vi "Interfaz grafica - corriente.vi"() -> ()   [LabVIEW 2024]
uses:
  160620 Optotune Lens Driver 4 Labview package/Hello Optotune Lens (30.06.2015)/Calibration.ctl
  <vilib>/DAQmx/read.llb/DAQmx Read (Analog 1D Wfm NChan NSamp).vi
  <vilib>/Analysis/2dsp.llb/Decimate (single shot, DBL).vi
  <vilib>/Utility/file.llb/Read Delimited Spreadsheet (string).vi
  <vilib>/Instr/_visa.llb/VISA Configure Serial Port (Instr).vi
  <vilib>/DAQmx/create/channels.llb/DAQmx Create Channel (AI-Voltage-Basic).vi
  <vilib>/DAQmx/configure/timing.llb/DAQmx Timing (Sample Clock).vi
  <vilib>/DAQmx/miscellaneous.llb/DAQmx Fill In Error Info.vi
  <vilib>/Waveform/WDTOps.llb/WDT Index Channel DBL.vi
  <vilib>/Analysis/2dsp.llb/Decimate (continuous, DBL).vi
  <vilib>/Utility/file.llb/Write Delimited Spreadsheet (string).vi
  <vilib>/Waveform/WDTOps.llb/WDT Get Waveform Time Array DBL.vi
  <vilib>/Analysis/NI_AALPro.lvlib
panel:
  out "Array 4":string[](array[string])
  out "Array 3":string[](array[string])
  out "Array 2":string[](array[string])
  out "Array":string[](array[string])
  out "Nombre 2":string
  in  "Restablecer Iniciales":bool
  in  "Incremento":dbl=0.1 format="%#_13g"
  out "Potencia derecho":dbl
  out "error out 4":errorcluster
  out "error out 3":errorcluster
  out "error out 2":errorcluster
  in  "Tab Control 3":enum32{"WL", "Video"}(tab)
  out "Waveform length":dbl[][](graph)
  in  "Minimo escala Y":dbl format="%#_13g"
  in  "Maximo escala Y":dbl format="%#_13g"
  in  "Escala autom. Y":u8=1
  in  "Escala autom. X":u8=1
  in  "Maximo escala X":dbl
  in  "Minimo escala X":dbl
  out "VISA resource name out":string
  in  "Tab Control 2":T1(tab)
  in  "DAQmx Physical Channel":tag
  in  "Frecuencia muestreo":i32=20000
  in  "tamaño buffer":i32=1000
  in  "factor decimacion":i32=20
  in  "Ganancia":u16(ring) items=["0.2"=51455, "1"=33023, "10"=49407, "20"=41215, "30"=57599, "40"=37119, "60"=53503, "80"=45311, "120"=61695, "157"=35071, ""=0]
  in  "Potencia inicial lente derecho":dbl(slide) scale=-3.0..3.0
  in  "Potencia inicial lente izquierdo":dbl(slide) scale=-3.0..3.0
  in  "VISA resource name":string="COM11"
  in  "VISA resource name 2":string="COM10"
  out "DPT INICIALES D":dbl
  out "DPT INICIALES I":dbl
  out "Potencia izquierdo":dbl
  in  "error in (no error) 5":errorcluster
  in  "error in (no error) 4":errorcluster
  in  "error in (no error) 3":errorcluster
  in  "error in (no error) 2":errorcluster
  in  "Calibration 4":T2={"Max Current A"=293.0, "Max Current B"=293.0, "UCL A"=300.0, "UCL B"=300.0, "LCL A"=0.0, "LCL B"=0.0} {"Max Current A" format="%#_g mA"; "Max Current B" format="%#_g mA"; "UCL A" format="%#_g mA"; "LCL A" format="%#_g mA"; "UCL B" format="%#_g mA"; "LCL B" format="%#_g mA"}
  out "ID 2":u16
  out "VISA resource name out 2":string
  out "Calibration 3":T2 {"Max Current A" format="%#_g mA"; "Max Current B" format="%#_g mA"; "UCL A" format="%#_g mA"; "LCL A" format="%#_g mA"; "UCL B" format="%#_g mA"; "LCL B" format="%#_g mA"}
  out "OK 2":bool
  out "Data 2":string
  out "Command to Port 2":string
  in  "Cola tipo 2":dbl[](array[numeric])
  in  "Tamaño ventana WL":i32=60
  in  "Limite inferior WL":dbl=25.0 format="%#_13g"
  in  "Limite superior WL":dbl=50.0
  out "number":u32
  in  "Calibration":T2={"Max Current A"=293.0, "Max Current B"=293.0, "UCL A"=300.0, "UCL B"=300.0, "LCL A"=0.0, "LCL B"=0.0} {"Max Current A" format="%#_g mA"; "Max Current B" format="%#_g mA"; "UCL A" format="%#_g mA"; "LCL A" format="%#_g mA"; "UCL B" format="%#_g mA"; "LCL B" format="%#_g mA"}
  out "ID":u16
  out "Calibration 2":T2 {"Max Current A" format="%#_g mA"; "Max Current B" format="%#_g mA"; "UCL A" format="%#_g mA"; "LCL A" format="%#_g mA"; "UCL B" format="%#_g mA"; "LCL B" format="%#_g mA"}
  out "OK":bool
  out "Data":string
  out "Command to Port":string
  in  "DPT dif.":dbl
  out "error out":errorcluster
  in  "error in (no error)":errorcluster
  in  "WL":dbl
  in  "Cola tipo":dbl[](array[numeric])
  out "T button?":bool
  in  "Elegir menu Exp":bool
  in  "Elegir menu":bool
  out "path":path
  in  "Iniciar experimento":bool
  in  "Parar adquisicion":bool
  out "Enfermedad visual":string
  out "Edad":string
  out "Nombre":string
  out "Cedula":string
  in  "Carpeta":path=path "C:/Users/TGM1603/Documents/LabVIEW Data/Experimentos electrodos"
  in  "?":bool
  in  "Menu Principal":u16(ring) items=["Visualizacion general ", "Llevar a cabo un experimento", "Ajustar potencia inicial lentes"]
  in  "Menu experimentos":u16(ring) items=["Experimento 1", "Experimento 2", "Experimento 3", "Experimento 4"]
  in  "Tab Control":enum32{"Señal EMG", "Potencia "}(tab)
  out "Senal EMG":waveform(dbl)[](graph)
  in  "Escala automatica Y":u8
  in  "Escala automatica X":u8=1
  in  "X Scale.Range:Increment":dbl
  in  "X Scale.Range:Minimum":dbl
  in  "X Scale.Range:Maximum":dbl
  in  "Y Scale.Range:Minimum":dbl=-5.0
  in  "Y Scale.Range:Maximum":dbl=5.0
  in  "Escala Y min":dbl
  in  "Escala Y max":dbl
  in  "Auto scale Y":u8=1
  in  "Escala X max":dbl
  in  "Escala X min":dbl
  out "Potencia Optica":dbl[](graph)
  in  "Auto scale X":u8=1
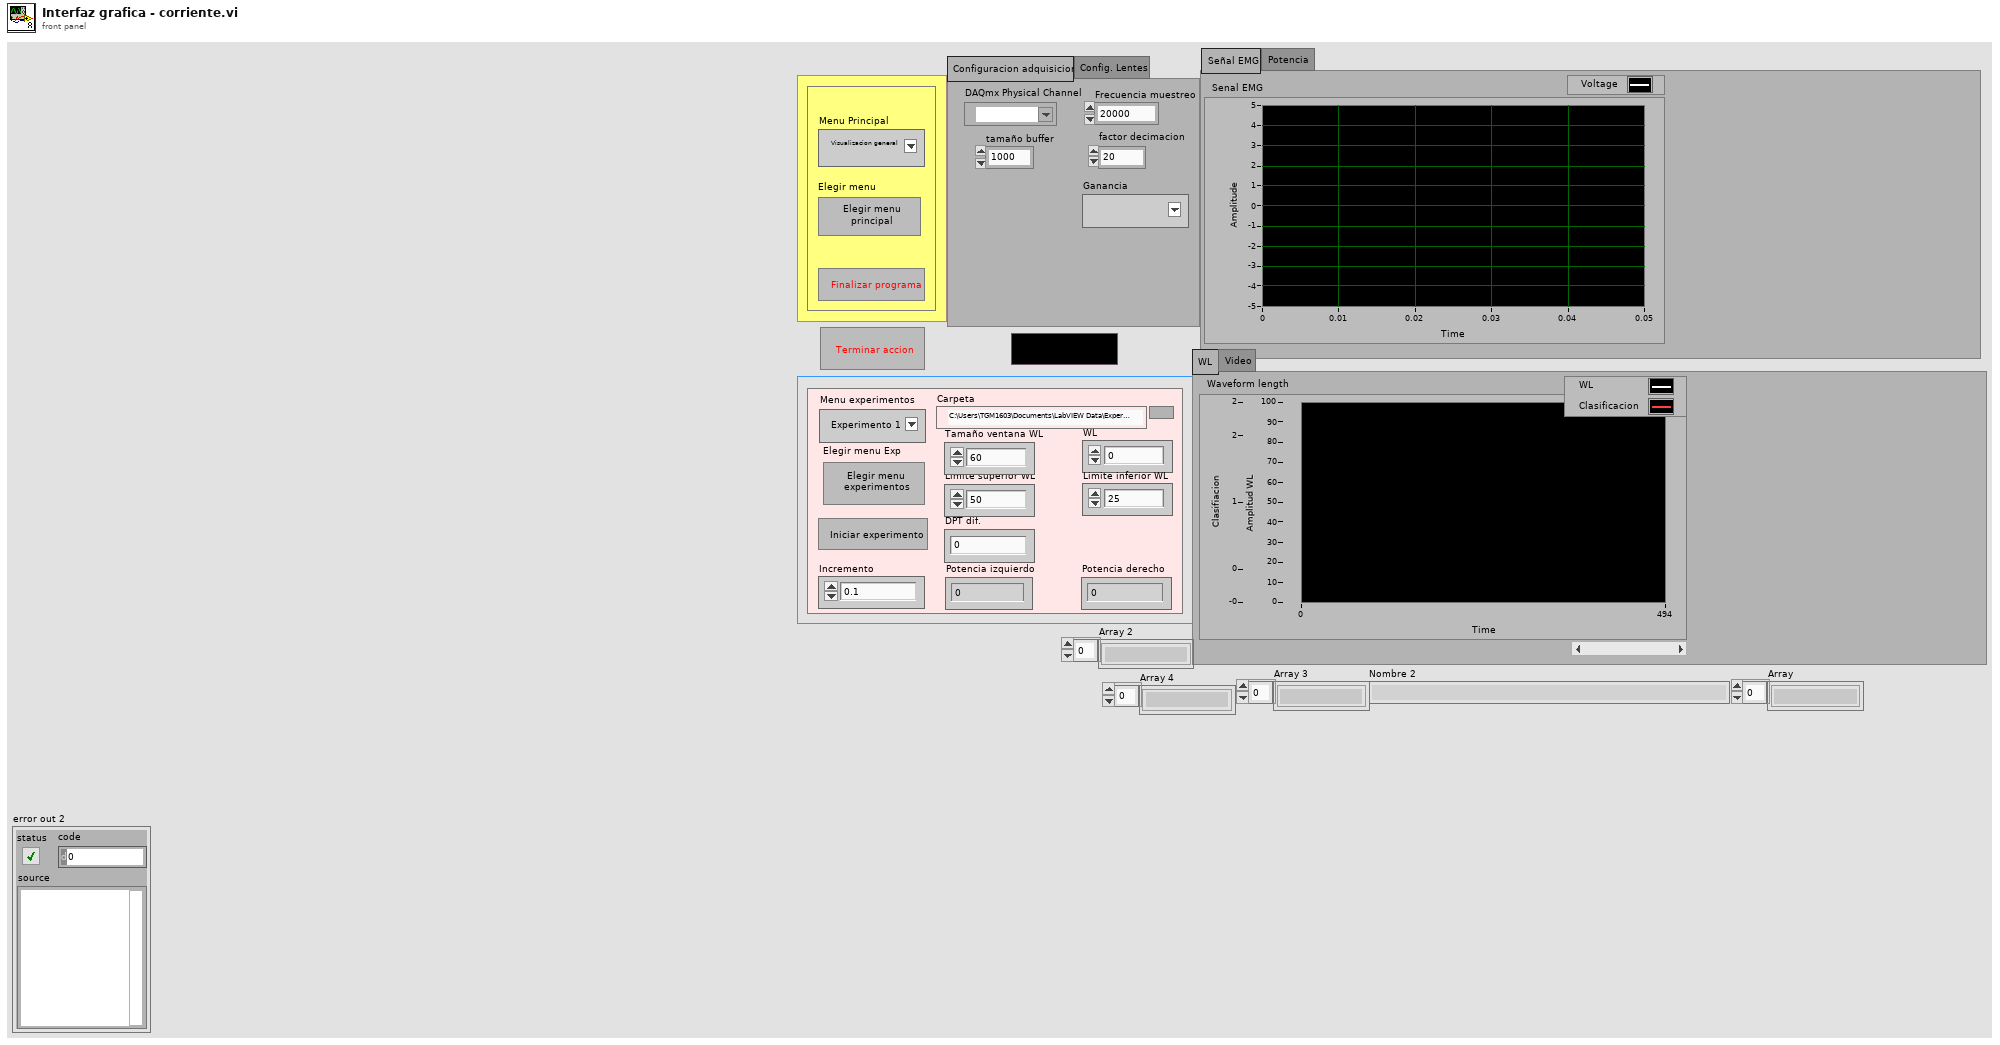
[diagram p1: front panel]
types:
  T1 = enum32{"Configuracion adquisicion", "Config. Lentes"}
  T2 = typedef "Calibration.ctl" = cluster{"Max Current A":dbl, "Max Current B":dbl, "UCL A":dbl, "UCL B":dbl, "LCL A":dbl, "LCL B":dbl}
  T3 = enum16{"Left Button", "Center Button", "Right Button", "Window Close"}
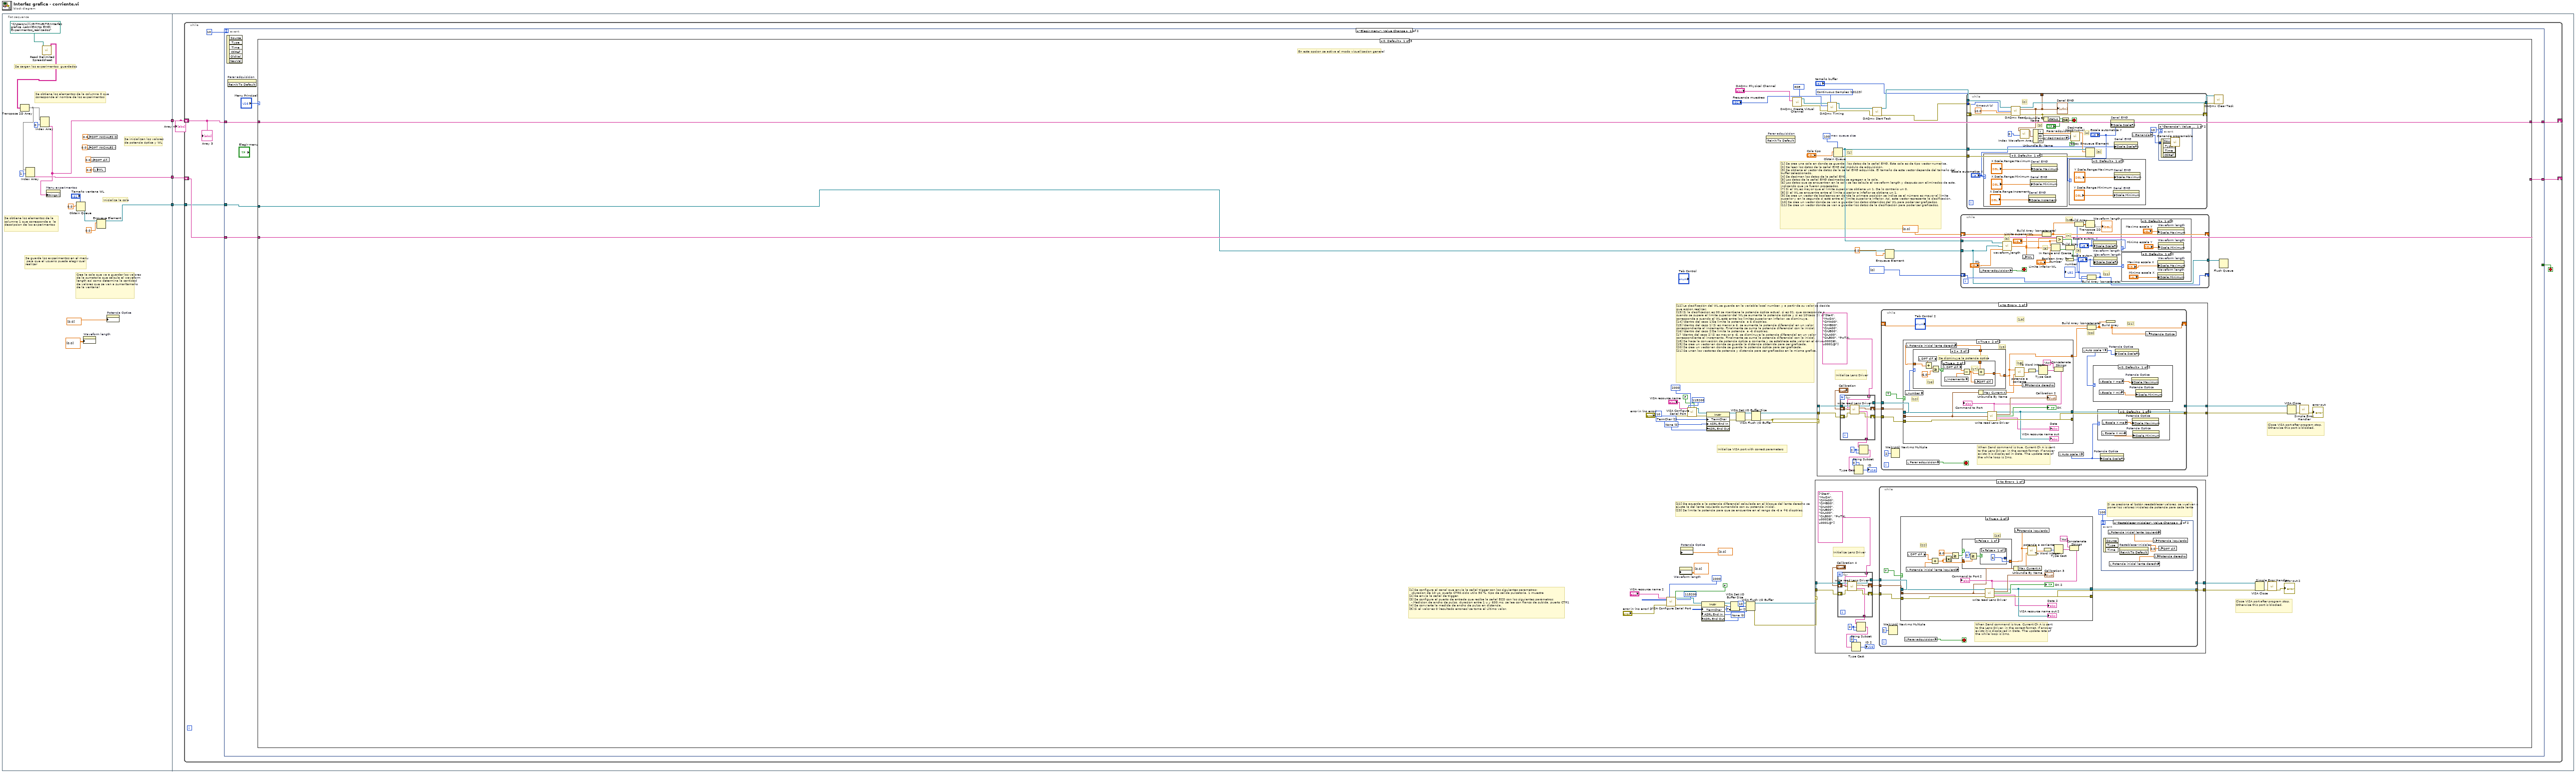
[diagram p0: block diagram]
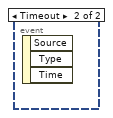
[diagram p2: hidden frame]
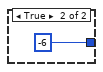
[diagram p4: hidden frame]
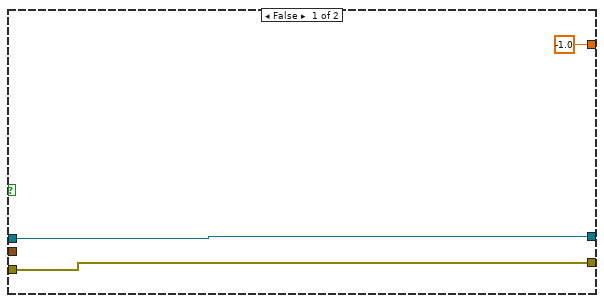
[diagram p9: hidden frame]
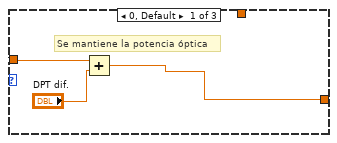
[diagram p10: hidden frame]
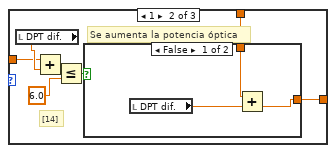
[diagram p11: hidden frame]
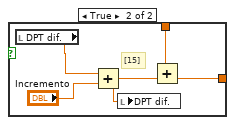
[diagram p12: hidden frame]
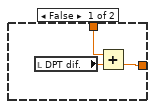
[diagram p13: hidden frame]
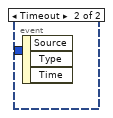
[diagram p17: hidden frame]
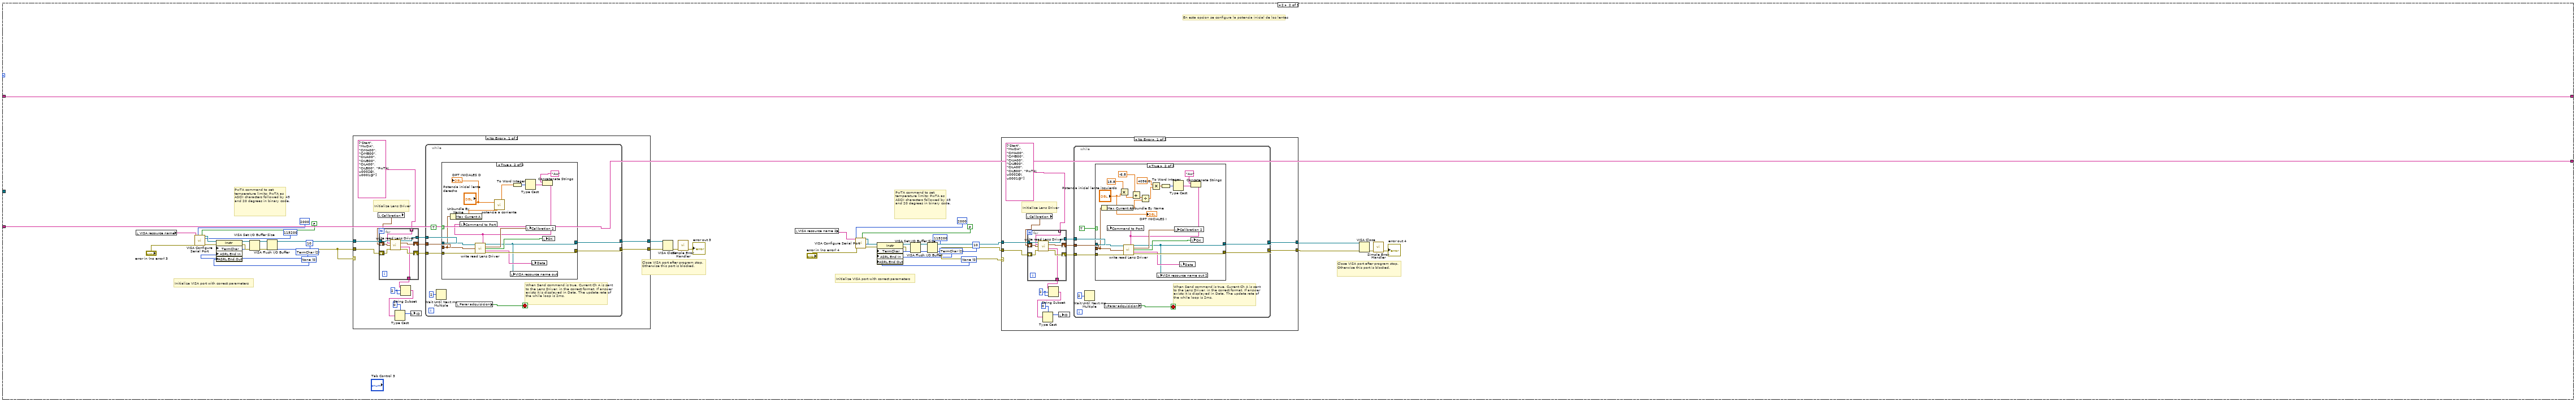
[diagram p20: hidden frame]
diagram:
  n1 = flat-sequence {
    tunnel: [w18] -> w3
    tunnel: [w15] -> w2
    tunnel: [w10] -> w1
    tunnel: w3 -> [w22]
    tunnel: w2 -> [w24]
    tunnel: w1 -> [w23]
    frame #0 {
      # "Se inicializan los valores\nde potencia óptica y WL"
      # "Inicializa la cola"
      # "Crea la cola que va a guardar los valores de la sumatoria que calcula el waveform length así como determina la cantidad de valores que se van a sumar(tamaño de la ventana)"
      # "Se obtiene los elementos de la columna 1 que corresponde a  la descripcion de los experimentos"
      # "Se obtiene los elementos de la columna 0 que corresponde al nombre de los experimentos"
      # "Se guarda los experimentos en el menu\n para que el usuario pueda elegir cual \nrealizar"
      # "Se cargan los experimentos  guardados"
      n2 = call-poly <vilib>:"Read Delimited Spreadsheet.vi"("file path (dialog if empty)"=path "C:/Users/willi/GITHUB/TG/Interfaz grafica -LabVIEW/No EMG/Experimentos_realizados") -> ("all rows"=w19:string[][])  [unwired: 9 in, 5 out]
      n3 = Transpose 2D Array(2D array=w19) -> (transposed array=w16:string[][])
      n4 = Index Array(array=w16, index (row)=1) -> (element=w15:string[])  [unwired: 1 in]
      n5 = Index Array(array=w16, index (row)=0) -> (element=w18:string[])  [unwired: 1 in]
      n6 = property on="Menu experimentos" class="Ring (strict)"("Strings []"=w18) -> ()  [unwired: 2 in, 2 out]
      n7 = Obtain Queue(max queue size (-1, unlimited)="Tamaño ventana WL", element data type=0.0) -> (queue out=w13:refnum<queue>)  [unwired: 3 in, 2 out]
      n8 = property on="Waveform length" class="WFChart (strict)"("History Data"=dbl[][] [[0.0]]) -> ()  [unwired: 2 in, 2 out]
      n9 = local write "DPT INICIALES D"(0.0 ("DPT INIT.1")) -> ()
      n10 = local write "DPT INICIALES I"(0.0 ("DPT INIT.2")) -> ()
      n11 = local write "DPT dif."(0.0 ("WL")) -> ()
      n12 = local write "WL"(0.0 ("WL")) -> ()
      n13 = Enqueue Element(queue=w13, element=0.0) -> (queue out=w10:refnum<queue>)  [unwired: 2 in, 2 out]
      n14 = property on="Potencia Optica" class="WFChart (strict)"("History Data"=dbl[] [0.0]) -> ()  [unwired: 2 in, 2 out]
    }
    frame #1 {
      n15 = while {
        shift-right: [w30] -> _
        shift-left: w22 -> [w31]
        shift-right: [w28] -> _
        shift-left: w24 -> [w29]
        tunnel: w23 -> [w27]
        stop <- w26 stop-if-true
        n16 = event shown="[0] \"Elegir menu\": Value Change" {
          selector: _ -> [_ _]
          dyn-events: _ -> [_ _]
          timeout: 10 -> [_ _]
          tunnel: w31 -> [w37 w978]
          tunnel: [w36 w978] -> w30
          tunnel: w29 -> [w35 w977]
          tunnel: [w34 w977] -> w28
          tunnel: w27 -> [w32 _]
          tunnel: [_ "?"] -> w26
          event "Elegir menu": Value Change {
            n17 = event-data() -> ()  [unwired: 1 in, 6 out]
            n18 = invoke on="Parar adquisicion" class="Bool (strict)" method="Reinit To Default"() -> ()  [unwired: 3 in, 3 out]
            n19 = case shown="0, Default" "Menu Principal" {
              tunnel: w37 -> [w104 w357 w477]
              tunnel: [w104 w357 w476] -> w36
              tunnel: w35 -> [w103 w356 w474]
              tunnel: [w103 w356 w473] -> w34
              tunnel: w32 -> [w93 _ w464]
              frame 0, Default {
                w38 = 10123 items=["Finite Samples"=10178, "Continuous Samples"=10123, "Hardware Timed Single Point"=12522] ("sample mode")
                w39 = 10083 items=["Default"=-1, "RSE"=10083, "NRSE"=10078, "Differential"=10106, "Pseudodifferential"=12529] ("input terminal configuration")
                w61 = u16 0 items=["None", "Last Bit", "TermChar", "Break"] ("Serial Settings:End Mode for Writes")
                w60 = u16 2 items=["None", "Last Bit", "TermChar"] ("Serial Settings:End Mode for Reads")
                w83 = u16 0 items=["None", "Last Bit", "TermChar", "Break"] ("Serial Settings:End Mode for Writes")
                w84 = u16 2 items=["None", "Last Bit", "TermChar"] ("Serial Settings:End Mode for Reads")
                w97 = 100  # max queue size
                # "[22] De acuerda a la potencia diferencial calculada en el bloque del lente derecho se ajusta la del lente izquierdo sumandola con su potencia inicial.\n[23] Se limita la potencia para que se encuentre en el rango de -6 a +6 dioptrías."
                # "[12] La clasificación del WL se guarda en la variable local number, y a partir de su valor se decide que accion realizar.\n[13] Si la clasificacion es 00 se mantiene la potencia óptica actual, si es 01, que corresponde a cuando se supera el limite superior del WL,se aumenta la potencia óptica y si es 10(caso 2), que corresponde a cuando el WL está entre los limites superior en inferior, se disminuye. \n[14] (dentro del caso 1)Se limita la potencia  a 6 dioptrías. \n[15] (dentro del caso 1) Si es menor a 6, se aumenta la potencia diferencial en un valor correspondiente al incremento. Finalmente se suma la potencia diferencial con la inicial.\n[16] (dentro del caso 2)Se limita la potencia  a -6 dioptrías.\n[17 (dentro del caso 2) Si es mayor a -6, se disminuye la potencia diferencial en un valor correspondiente al incremento. Finalmente se suma la potencia diferencial con la inicial.\n[18] Se hace la conversión de potencia óptica a corriente y se establece este valor en el driver.\n[19] Se crea un vector en donde se guarda la distancia obtenida para ser graficada.\n[20] Se crea un vector en donde se guarda la potencia óptica para ser graficada.\n[21] Se unen los vectores de potencia y distancia para ser graficados en la misma grafica."
                # "[1] Se crea una cola en donde se guardan los datos de la señal EMG. Esta cola es de tipo vector numerica.\n[2] Se leen los datos de la señal EMG del módulo de adquisición. \n[3] Se obtiene el vector de datos de la señal EMG adquirida. El tamaño de este vector depende del tamaño del buffer seleccionado.\n[4] Se deciman los datos de la señal EMG.\n[5] Los datos de la señal EMG decimados se agregan a la cola.\n[6] Los datos que se encuentran en la cola se les calcula el waveform length y después son eliminados de esta, indicando que ya fueron procesados. \n[7] Si el WL es mayor que el limite superior se obtiene un 1. De lo contrario un 0.\n[8] Si el WL se encuentra entre el límite superior e infefior se obtiene un 1.\n[9] Se crea un vector de booleanos en donde la primera posición se indica se el número es mayor al límite superior y en la segunda si está entre el  limite superior e inferior. Así, este vector representa la clasificación.\n[10] Se crea un vector donde se van a guardar los datos obtenidos del WL para poder ser graficados.\n[11] Se crea un vector donde se van a guardar los datos de la clasificación para poder ser graficados."
                # "[1]"
                # "En esta opcion se activa el modo visualizacion general"
                # "Close VISA port after program stop. Otherwise this port is blocked."
                # "[1] Se configura el canal que envía la señal trigger con los siguientes parametros:\n  -duracion de 10 us, puerto CTR0,ciclo utilo 50 %, tipo de salida pulsatoria, 1 muestra \n[2] Se envía la señal de trigger.\n[3] Se configura el puerto de entrada que recibe la señal ECO con los siguientes parámetros:\n  - Medicion de ancho de pulso, duracion entre 1 u y 600 ms, se lee con flanco de subida, puerto CTR1\n[4] Se convierte la medida de ancho de pulso en distancia.\n[5] Si el valor es 0 (resultado erroneo) se toma el último valor."
                # "Close VISA port after program stop. Otherwise this port is blocked."
                # "Initialize VISA port with correct parameters"
                n20 = call-poly "VISA Configure Serial Port"("VISA resource name"="VISA resource name 2", "timeout (10sec)"=u32 2000, "Enable Termination\nChar (T)"=FALSE ("Enable Termination\nChar (T)"), "baud rate (9600)"=u32 115200, "error in (no error)"="error in (no error) 2") -> ("VISA resource name out"=w56:refnum<visa-resource-name>, "error out"=w58:errorcluster)  [unwired: 9 in]
                n21 = property on="Waveform length" class="WFChart (strict)"("History Data"=dbl[][] [[0.0]]) -> ()  [unwired: 2 in, 2 out]
                n22 = property on="Potencia Optica" class="WFChart (strict)"("History Data"=dbl[] [0.0]) -> ()  [unwired: 2 in, 2 out]
                n23 = call-poly "VISA Configure Serial Port"("VISA resource name"="VISA resource name", "timeout (10sec)"=u32 2000, "Enable Termination\nChar (T)"=FALSE ("Enable Termination\nChar (T)"), "baud rate (9600)"=u32 115200, "error in (no error)"="error in (no error)") -> ("VISA resource name out"=w88:refnum<visa-resource-name>, "error out"=w86:errorcluster)  [unwired: 9 in]
                n24 = property class="Instr"(reference=w56, error in=w58, "TermChar"=u8 10 ("Message Based Settings:Termination Character"), "ASRL End In"=w60, "ASRL End Out"=w61) -> (reference out=w57:refnum<visa-resource-name>, error out=w59:errorcluster)
                n25 = property class="Instr"(reference=w88, error in=w86, "TermChar"=u8 10 ("Message Based Settings:Termination Character"), "ASRL End In"=w84, "ASRL End Out"=w83) -> (reference out=w87:refnum<visa-resource-name>, error out=w85:errorcluster)
                n26 = VISA Set I/O Buffer Size(VISA resource name=w57, error in (no error)=w59) -> (VISA resource name out=w64:refnum<visa-resource-name>, error out=w65:errorcluster)  [unwired: 2 in]
                n27 = VISA Set I/O Buffer Size(VISA resource name=w87, error in (no error)=w85) -> (VISA resource name out=w80:refnum<visa-resource-name>, error out=w79:errorcluster)  [unwired: 2 in]
                n28 = VISA Flush I/O Buffer(VISA resource name=w64, error in (no error)=w65) -> (VISA resource name out=w50:refnum<visa-resource-name>, error out=w51:errorcluster)  [unwired: 1 in]
                n29 = VISA Flush I/O Buffer(VISA resource name=w80, error in (no error)=w79) -> (VISA resource name out=w78:refnum<visa-resource-name>, error out=w73:errorcluster)  [unwired: 1 in]
                n30 = invoke on="Parar adquisicion" class="Bool (strict)" method="Reinit To Default"() -> ()  [unwired: 3 in, 3 out]
                n31 = call-poly <vilib>:"DAQmx Create Virtual Channel.vi"("input terminal configuration"=w39, "physical channels"="DAQmx Physical Channel") -> ("task out"=w45:refnum<k21>, "error out"=w44:errorcluster)  [unwired: 12 in]
                n32 = case shown="No Error" w51 {
                  tunnel: w51 -> [w118 w169]
                  tunnel: w50 -> [w117 w170]
                  tunnel: [w116 w169] -> w46
                  tunnel: [w115 w170] -> w47
                  frame No Error {
                    w113 = 2 ("length (rest)")
                    # "Initialize Lens Driver"
                    n33 = for {
                      tunnel: w117 -> [w167]
                      tunnel: [w164] -> w107
                      tunnel: string[] ["Start", "MwDA", "CrMA00", "CrMB00", "CrUA00", "CrUB00", "CrLA00", "CrLB00", "PwTA\u0002Ð\u0001@"] -> [w162] mode=indexing
                      tunnel: [w161] -> w106
                      shift-right: [w165] -> w108
                      shift-left: "Calibration 4" -> [w166]
                      shift-right: [w163] -> w109
                      shift-left: w118 -> [w168]
                      n34 = call "write read Lens Driver.vi"("VISA resource name"=w167, "command"=w162, "Calibration"=w166, "error in (no error)"=w168) -> ("VISA resource name out"=w164:refnum<visa-resource-name>, "Calibration 2"=w165:T2, "Data"=w161:string, "error out"=w163:errorcluster)  [unwired: 4 in, 4 out]
                    }
                    n35 = String Subset(string=w106, offset (0)=w113, length (rest)=w113) -> (substring=w111:string)
                    n36 = Type Cast(type=u16 0 ("length (rest)"), x=w111) -> (*(type *) &x=→"ID 2":u16)
                    n37 = while {
                      tunnel: [w121] -> w116
                      tunnel: [w122] -> w115
                      tunnel: w109 -> [w127]
                      tunnel: w108 -> [w126]
                      tunnel: w107 -> [w125]
                      stop <- w120 stop-if-true
                      # "Si se presiona el botón reestablecer valores, se vuelven a poner los valores iniciales de potencia para cada lente"
                      # "When Send command is true, Current Ch A is sent to the Lens Driver, in the correct format. If answer exists it is displayed in Data. The update rate of the while loop is 2ms."
                      n38 = Wait Until Next ms Multiple(millisecond multiple=u32 2) -> ()  [unwired: 1 out]
                      n39 = case shown="True" TRUE ("Send command") {
                        tunnel: [w132 w153] -> w121
                        tunnel: w127 -> [w132 w152]
                        tunnel: w126 -> [_ w134]
                        tunnel: w125 -> [w131 w151]
                        tunnel: [w131 w148] -> w122
                        frame False {
                        }
                        frame True {
                          # "[23]"
                          # "[22]"
                          n40 = local read "Potencia inicial lente izquierdo"() -> (w142:dbl)
                          n41 = local read "DPT dif."() -> (w143:dbl)
                          n42 = Add(x=w143, y=w142) -> (x+y=w138:dbl)
                          n43 = Absolute Value(x=w138) -> (abs(x)=w140:dbl)
                          n44 = Greater Or Equal?(x=6.0, y=w140) -> (x >= y?=w141:bool)
                          n45 = case shown="False" w141 {
                            tunnel: w138 -> [w156 w160]
                            tunnel: [w154 w160] -> w136
                            frame False {
                              n46 = Greater Or Equal?(x=u16 0, y=w156) -> (x >= y?=w157:bool)
                              n47 = case shown="False" w157 {
                                tunnel: [i16 6 ("x") i16 -6 ("x")] -> w154
                                frame False {
                                }
                                frame True {
                                }
                              }
                            }
                            frame True {
                            }
                          }
                          n48 = Unbundle By Name(w134) -> ("Max Current A"=w135:dbl)
                          n49 = local write "Potencia izquierdo"(w136) -> ()
                          n50 = call "potencia a corriente.vi"("Max current A"=w135, "Potencia"=w136) -> ("Corriente"=w137:dbl)
                          n51 = To Word Integer(number=w137) -> (16bit integer=w146:i16)
                          n52 = Type Cast(x=w146) -> (*(type *) &x=w145:string)  [unwired: 1 in]
                          n53 = Concatenate Strings("Aw", w145) -> (w144:string)
                          "Command to Port 2" <- w144
                          n54 = call "write read Lens Driver.vi"("VISA resource name"=w151, "command"=w144, "Calibration"=w134, "error in (no error)"=w152) -> ("VISA resource name out"=w148:refnum<visa-resource-name>, "Calibration 2"=→"Calibration 3":T2, "OK"=→"OK 2":bool, "Data"=→"Data 2":string, "error out"=w153:errorcluster)  [unwired: 4 in, 3 out]
                          "VISA resource name out 2" <- w148
                        }
                      }
                      n55 = local read "Parar adquisicion"() -> (w120:bool)
                      n56 = event shown="[0] \"Restablecer Iniciales\": Value Change" {
                        selector: _ -> [_ _]
                        dyn-events: _ -> [_ _]
                        timeout: 100 -> [_ _]
                        event "Restablecer Iniciales": Value Change {
                          n57 = event-data() -> ()  [unwired: 1 in, 3 out]
                          n58 = local read "Potencia inicial lente izquierdo"() -> (w128:dbl)
                          n59 = local read "Potencia inicial lente derecho"() -> (w129:dbl)
                          n60 = invoke on="Restablecer Iniciales" class="Bool" method="Reinit To Default"() -> ()  [unwired: 3 in, 3 out]
                          n61 = local write "Potencia izquierdo"(w128) -> ()
                          n62 = local write "Potencia derecho"(w129) -> ()
                          n63 = local write "DPT dif."(0.0 ("DPT dif.")) -> ()
                        }
                        event Timeout {
                          n64 = event-data() -> ()  [unwired: 1 in, 3 out]
                        }
                      }
                    }
                  }
                  frame Error {
                  }
                }
                n65 = case shown="No Error" w73 {
                  tunnel: w73 -> [w184 w263]
                  tunnel: w78 -> [w183 w264]
                  tunnel: [w182 w263] -> w76
                  tunnel: [w181 w264] -> w74
                  frame No Error {
                    w179 = 2 ("length (rest)")
                    # "Initialize Lens Driver"
                    n66 = for {
                      tunnel: w183 -> [w261]
                      tunnel: [w258] -> w173
                      tunnel: string[] ["Start", "MwDA", "CrMA00", "CrMB00", "CrUA00", "CrUB00", "CrLA00", "CrLB00", "PwTA\u0002Ð\u0001@"] -> [w256] mode=indexing
                      tunnel: [w255] -> w172
                      shift-right: [w259] -> w174
                      shift-left: "Calibration" -> [w260]
                      shift-right: [w257] -> w175
                      shift-left: w184 -> [w262]
                      n67 = call "write read Lens Driver.vi"("VISA resource name"=w261, "command"=w256, "Calibration"=w260, "error in (no error)"=w262) -> ("VISA resource name out"=w258:refnum<visa-resource-name>, "Calibration 2"=w259:T2, "Data"=w255:string, "error out"=w257:errorcluster)  [unwired: 4 in, 4 out]
                    }
                    n68 = String Subset(string=w172, offset (0)=w179, length (rest)=w179) -> (substring=w177:string)
                    n69 = Type Cast(type=u16 0 ("length (rest)"), x=w177) -> (*(type *) &x=→"ID":u16)
                    n70 = while {
                      tunnel: [w191] -> w182
                      tunnel: [w192] -> w181
                      tunnel: w175 -> [w197]
                      tunnel: w174 -> [w196]
                      tunnel: w173 -> [w195]
                      shift-right: [w185] -> _
                      shift-left: _ -> [w187]
                      stop <- w190 stop-if-true
                      # "[21]"
                      # "[20]"
                      # "[19]"
                      # "When Send command is true, Current Ch A is sent to the Lens Driver, in the correct format. If answer exists it is displayed in Data. The update rate of the while loop is 2ms."
                      n71 = Wait Until Next ms Multiple(millisecond multiple=u32 2) -> ()  [unwired: 1 out]
                      n72 = case shown="True" TRUE ("Send command") {
                        tunnel: [w204 w221] -> w191
                        tunnel: w197 -> [w204 w220]
                        tunnel: w196 -> [_ w207]
                        tunnel: w195 -> [w203 w219]
                        tunnel: [w203 w216] -> w192
                        tunnel: [-1.0 ("DPT") w209] -> w186
                        frame False {
                        }
                        frame True {
                          # "[18]"
                          # "[13]"
                          # "[12]"
                          n73 = local read "number"() -> (w211:u32)
                          n74 = local read "Potencia inicial lente derecho"() -> (w210:dbl)
                          n75 = case shown="2" w211 {
                            tunnel: [w223 w231 w246] -> w209
                            tunnel: w210 -> [w224 w226 w241]
                            tunnel: w210 -> [_ w225 w240]
                            frame 0, Default {
                              # "Se mantiene la potencia óptica"
                              n76 = Add(x=w224, y="DPT dif.") -> (x+y=w223:dbl)
                            }
                            frame 1 {
                              # "[14]"
                              # "Se aumenta la potencia óptica"
                              n77 = local read "DPT dif."() -> (w227:dbl)
                              n78 = Add(x=w226, y=w227) -> (x+y=w228:dbl)
                              n79 = Less Or Equal?(x=w228, y=6.0) -> (x <= y?=w230:bool)
                              n80 = case shown="False" w230 {
                                tunnel: [w233 w236] -> w231
                                tunnel: w225 -> [w232 w235]
                                frame False {
                                n81 = local read "DPT dif."() -> (w234:dbl)
                                n82 = Add(x=w232, y=w234) -> (x+y=w233:dbl)
                                }
                                frame True {
                                # "[15]"
                                n83 = local read "DPT dif."() -> (w237:dbl)
                                n84 = Add(x=w237, y="Incremento") -> (x+y=w238:dbl)
                                n85 = local write "DPT dif."(w238) -> ()
                                n86 = Add(x=w235, y=w238) -> (x+y=w236:dbl)
                                }
                              }
                            }
                            frame 2 {
                              # "[16]"
                              # "Se disminuye la potencia óptica"
                              n87 = local read "DPT dif."() -> (w245:dbl)
                              n88 = Add(x=w245, y=w241) -> (x+y=w242:dbl)
                              n89 = Greater Or Equal?(x=w242, y=-6.0) -> (x >= y?=w243:bool)
                              n90 = case shown="True" w243 {
                                tunnel: [w248 w252] -> w246
                                tunnel: w240 -> [w247 w251]
                                frame False {
                                n91 = local read "DPT dif."() -> (w249:dbl)
                                n92 = Add(x=w247, y=w249) -> (x+y=w248:dbl)
                                }
                                frame True {
                                # "[17]"
                                n93 = local read "DPT dif."() -> (w254:dbl)
                                n94 = local read "Incremento"() -> (w250:dbl)
                                n95 = Subtract(x=w254, y=w250) -> (x-y=w253:dbl)
                                n96 = local write "DPT dif."(w253) -> ()
                                n97 = Add(x=w251, y=w253) -> (x+y=w252:dbl)
                                }
                              }
                            }
                          }
                          n98 = Unbundle By Name(w207) -> ("Max Current A"=w206:dbl)
                          n99 = call "potencia a corriente.vi"("Max current A"=w206, "Potencia"=w209) -> ("Corriente"=w208:dbl)
                          n100 = local write "Potencia derecho"(w209) -> ()
                          n101 = To Word Integer(number=w208) -> (16bit integer=w214:i16)
                          n102 = Type Cast(x=w214) -> (*(type *) &x=w213:string)  [unwired: 1 in]
                          n103 = Concatenate Strings("Aw", w213) -> (w212:string)
                          "Command to Port" <- w212
                          n104 = call "write read Lens Driver.vi"("VISA resource name"=w219, "command"=w212, "Calibration"=w207, "error in (no error)"=w220) -> ("VISA resource name out"=w216:refnum<visa-resource-name>, "Calibration 2"=→"Calibration 2":T2, "OK"=→"OK":bool, "Data"=→"Data":string, "error out"=w221:errorcluster)  [unwired: 4 in, 3 out]
                          "VISA resource name out" <- w216
                        }
                      }
                      n105 = local read "Parar adquisicion"() -> (w190:bool)
                      n106 = local read "Auto scale X"() -> (w188:u8)
                      n107 = local read "Auto scale Y"() -> (w189:u8)
                      n108 = Build Array (concatenate)(w187, w186) -> (w185:dbl[])
                      n109 = case shown="0, Default" w189 {
                        frame 0, Default {
                          n110 = local read "Escala Y max"() -> (w201:dbl)
                          n111 = local read "Escala Y min"() -> (w200:dbl)
                          n112 = property on="Potencia Optica" class="WFChart (strict)"("YScale.Maximum"=w201) -> ()  [unwired: 2 in, 2 out]
                          n113 = property on="Potencia Optica" class="WFChart (strict)"("YScale.Minimum"=w200) -> ()  [unwired: 2 in, 2 out]
                        }
                        frame 1 {
                        }
                      }
                      n114 = case shown="0, Default" w188 {
                        frame 0, Default {
                          n115 = local read "Escala X min"() -> (w198:dbl)
                          n116 = local read "Escala X max"() -> (w199:dbl)
                          n117 = property on="Potencia Optica" class="WFChart (strict)"("XScale.Maximum"=w199) -> ()  [unwired: 2 in, 2 out]
                          n118 = property on="Potencia Optica" class="WFChart (strict)"("XScale.Minimum"=w198) -> ()  [unwired: 2 in, 2 out]
                        }
                        frame 1 {
                        }
                      }
                      n119 = property on="Potencia Optica" class="WFChart (strict)"("XScale.ScaleFit"=w188) -> ()  [unwired: 2 in, 2 out]
                      n120 = Build Array(w185) -> ()  [unwired: 1 out]
                      n121 = property on="Potencia Optica" class="WFChart (strict)"("YScale.ScaleFit"=w189) -> ()  [unwired: 2 in, 2 out]
                      n122 = local write "Potencia Optica"(w185) -> ()
                    }
                  }
                  frame Error {
                  }
                }
                n123 = call-poly <vilib>:"DAQmx Timing.vi"("task/channels in"=w45, "sample mode"=w38, "rate"="Frecuencia muestreo", "error in"=w44) -> ("task out"=w43:refnum<k21>, "error out"=w42:errorcluster)  [unwired: 10 in]
                n124 = Obtain Queue(max queue size (-1, unlimited)=w97, element data type="Cola tipo") -> (queue out=w94:refnum<queue>, error out=w95:errorcluster)  [unwired: 3 in, 1 out]
                n125 = call <vilib>:"DAQmx Start Task.vi"("task/channels in"=w43, "error in"=w42) -> ("task out"=w102:refnum<k21>, "error out"=w101:errorcluster)  [unwired: 12 in]
                n126 = Enqueue Element(queue=w93, element=0.0) -> (queue out=w70:refnum<queue>)  [unwired: 2 in, 2 out]
                n127 = while {
                  tunnel: w70 -> [w266]
                  tunnel: w94 -> [w283]
                  shift-right: [w269] -> _
                  shift-left: dbl[] [0.0] -> [w280]
                  shift-right: [w268] -> _
                  shift-left: u32[] [0] -> [w270]
                  tunnel: [w266] -> w68
                  stop <- w281 stop-if-true
                  # "[11]"
                  # "[10]"
                  # "[9]"
                  # "[8]"
                  # "[7]"
                  # "[6]"
                  n128 = local read "Parar adquisicion"() -> (w281:bool)
                  n129 = call "waveform_length.vi"("WL"="WL", "Cola WL"=w266, "Datos entrada"=w283) -> ("WL 2"=w278:dbl)
                  n130 = local write "WL"(w278) -> ()
                  n131 = Build Array (concatenate)(w280, w278) -> (w269:dbl[])
                  n132 = In Range and Coerce(upper limit="Limite superior WL", x=w278, lower limit="Limite inferior WL") -> (In Range?=w276:bool)  [unwired: 1 out]
                  n133 = Greater?(x=w278, y="Limite superior WL") -> (0:w277:bool)
                  n134 = Build Array(w277, w276) -> (w275:bool[])
                  n135 = Boolean Array To Number(Boolean array=w275) -> (number=w271:u32)
                  "number" <- w271
                  n136 = Build Array (concatenate)(w270, w271) -> (w268:u32[])
                  n137 = Build Array(w269, w268) -> (w267:dbl[][])
                  n138 = Transpose 2D Array(2D array=w267) -> (transposed array=→"Waveform length":dbl[][])
                  n139 = property on="Waveform length" class="WFChart (strict)"("YScale.ScaleFit"="Escala autom. Y") -> ()  [unwired: 2 in, 2 out]
                  n140 = property on="Waveform length" class="WFChart (strict)"("XScale.ScaleFit"="Escala autom. X") -> ()  [unwired: 2 in, 2 out]
                  n141 = case shown="0, Default" "Escala autom. Y" {
                    frame 0, Default {
                      n142 = property on="Waveform length" class="WFChart (strict)"("YScale.Maximum"="Maximo escala Y") -> ()  [unwired: 2 in, 2 out]
                      n143 = property on="Waveform length" class="WFChart (strict)"("YScale.Minimum"="Minimo escala Y") -> ()  [unwired: 2 in, 2 out]
                    }
                    frame 1 {
                    }
                  }
                  n144 = case shown="0, Default" "Escala autom. X" {
                    frame 0, Default {
                      n145 = property on="Waveform length" class="WFChart (strict)"("XScale.Minimum"="Minimo escala X") -> ()  [unwired: 2 in, 2 out]
                      n146 = property on="Waveform length" class="WFChart (strict)"("XScale.Maximum"="Maximo escala X") -> ()  [unwired: 2 in, 2 out]
                    }
                    frame 1 {
                    }
                  }
                }
                n147 = while {
                  tunnel: w102 -> [w309]
                  tunnel: "tamaño buffer" -> [w306]
                  tunnel: [w307] -> w98
                  shift-right: [w304] -> w99
                  shift-left: w101 -> [w308]
                  tunnel: [w298] -> _
                  tunnel: w94 -> [w294]
                  tunnel: w95 -> [w293]
                  stop <- w303 stop-if-true
                  w302 = 10.0  # timeout (s)
                  # "[5]"
                  # "[4]"
                  # "[3]"
                  # "[2]"
                  n148 = case shown="0, Default" "Escala automatica X" {
                    frame 0, Default {
                      n149 = property on="Senal EMG" class="WFGraph (strict)"("XScale.Increment"="X Scale.Range:Increment") -> ()  [unwired: 2 in, 2 out]
                      n150 = property on="Senal EMG" class="WFGraph (strict)"("XScale.Minimum"="X Scale.Range:Minimum") -> ()  [unwired: 2 in, 2 out]
                      n151 = property on="Senal EMG" class="WFGraph (strict)"("XScale.Maximum"="X Scale.Range:Maximum") -> ()  [unwired: 2 in, 2 out]
                    }
                    frame 1 {
                    }
                  }
                  n152 = call-poly <vilib>:"DAQmx Read.vi"("task/channels in"=w309, "number of samples per channel"=w306, "timeout"=w302, "error in"=w308) -> ("task out"=w307:refnum<k21>, "data"=w298:waveform(dbl)[], "error out"=w304:errorcluster)  [unwired: 9 in]
                  "Senal EMG" <- w298
                  n153 = call-poly <vilib>:"Index Waveform Array.vi"("index"=0, "waveform array"=w298) -> ("waveform"=w299:waveform(dbl))  [unwired: 8 in, 1 out]
                  n154 = Unbundle By Name(w299) -> ("Y"=w296:dbl[])  [unwired: 2 out]
                  n155 = local read "factor decimacion"() -> (w295:i32)
                  n156 = Unbundle By Name(w304) -> ("status"=w305:bool)
                  n157 = Or(x=w305, y="Parar adquisicion") -> (x .or. y?=w303:bool)
                  n158 = case shown="0, Default" "Escala automatica Y" {
                    frame 0, Default {
                      n159 = property on="Senal EMG" class="WFGraph (strict)"("YScale.Minimum"="Y Scale.Range:Minimum") -> ()  [unwired: 2 in, 2 out]
                      n160 = property on="Senal EMG" class="WFGraph (strict)"("YScale.Maximum"="Y Scale.Range:Maximum") -> ()  [unwired: 2 in, 2 out]
                    }
                    frame 1 {
                    }
                  }
                  n161 = call-poly <vilib>:"Decimate (continuous).vi"("averaging"=TRUE, "decimating factor"=w295, "X"=w296) -> ("Decimated Array"=w292:dbl[])  [unwired: 7 in, 1 out]
                  n162 = Lossy Enqueue Element(queue=w294, element=w292, error in (no error)=w293) -> ()  [unwired: 4 out]
                  n163 = property on="Senal EMG" class="WFGraph (strict)"("YScale.ScaleFit"="Escala automatica Y") -> ()  [unwired: 2 in, 2 out]
                  n164 = property on="Senal EMG" class="WFGraph (strict)"("XScale.ScaleFit"="Escala automatica X") -> ()  [unwired: 2 in, 2 out]
                  n165 = local read "Ganancia"() -> (w289:u16)
                  n166 = event shown="[0] \"Ganancia\": Value Change" {
                    selector: _ -> [_ _]
                    dyn-events: _ -> [_ _]
                    timeout: 10 -> [_ _]
                    tunnel: w289 -> [w310 _]
                    event "Ganancia": Value Change {
                      n167 = event-data() -> ()  [unwired: 1 in, 4 out]
                      n168 = call "Ganancia programable.vi"("MOSI data"=w310) -> ()
                    }
                    event Timeout {
                      n169 = event-data() -> ()  [unwired: 1 in, 3 out]
                    }
                  }
                }
                n170 = call <vilib>:"DAQmx Clear Task.vi"("task in"=w98, "error in"=w99) -> ()  [unwired: 13 in, 1 out]
                n171 = Flush Queue(queue=w68) -> ()  [unwired: 1 in, 3 out]
                n172 = VISA Close(VISA resource name=w47, error in (no error)=w46) -> (error out=w48:errorcluster)
                n173 = call <vilib>:"Simple Error Handler.vi"("error in (no error)"=w48) -> ("error out"=→"error out 2":errorcluster)  [unwired: 4 in, 4 out]
                n174 = VISA Close(VISA resource name=w74, error in (no error)=w76) -> (error out=w77:errorcluster)
                n175 = call <vilib>:"Simple Error Handler.vi"("error in (no error)"=w77) -> ("error out"=→"error out":errorcluster)  [unwired: 4 in, 4 out]
              }
              frame 2 {
                w336 = u16 0 items=["None", "Last Bit", "TermChar", "Break"] ("Serial Settings:End Mode for Writes")
                w335 = u16 2 items=["None", "Last Bit", "TermChar"] ("Serial Settings:End Mode for Reads")
                w349 = u16 0 items=["None", "Last Bit", "TermChar", "Break"] ("Serial Settings:End Mode for Writes")
                w348 = u16 2 items=["None", "Last Bit", "TermChar"] ("Serial Settings:End Mode for Reads")
                # "En esta opcion se configura la potencia inicial de los lentes"
                # "Close VISA port after program stop. Otherwise this port is blocked."
                # "Close VISA port after program stop. Otherwise this port is blocked."
                # "PwTA command to set temperature limits: PwTA as ASCII characters followed by 45 and 20 degrees in binary code."
                # "Initialize VISA port with correct parameters"
                # "PwTA command to set temperature limits: PwTA as ASCII characters followed by 45 and 20 degrees in binary code."
                # "Initialize VISA port with correct parameters"
                n176 = local read "VISA resource name"() -> (w326:string)
                n177 = call-poly "VISA Configure Serial Port"("VISA resource name"=w326, "timeout (10sec)"=u32 2000, "Enable Termination\nChar (T)"=FALSE ("Enable Termination\nChar (T)"), "baud rate (9600)"=u32 115200, "error in (no error)"="error in (no error) 3") -> ("VISA resource name out"=w331:refnum<visa-resource-name>, "error out"=w333:errorcluster)  [unwired: 9 in]
                n178 = property class="Instr"(reference=w331, error in=w333, "TermChar"=u8 10 ("Message Based Settings:Termination Character"), "ASRL End In"=w335, "ASRL End Out"=w336) -> (reference out=w332:refnum<visa-resource-name>, error out=w334:errorcluster)
                n179 = VISA Set I/O Buffer Size(VISA resource name=w332, error in (no error)=w334) -> (VISA resource name out=w338:refnum<visa-resource-name>, error out=w339:errorcluster)  [unwired: 2 in]
                n180 = VISA Flush I/O Buffer(VISA resource name=w338, error in (no error)=w339) -> (VISA resource name out=w325:refnum<visa-resource-name>, error out=w324:errorcluster)  [unwired: 1 in]
                n181 = case shown="No Error" w324 {
                  tunnel: w324 -> [w371 w405]
                  tunnel: w325 -> [w370 w406]
                  tunnel: [w369 w405] -> w320
                  tunnel: [w368 w406] -> w321
                  frame No Error {
                    w367 = 2 ("length (rest)")
                    # "Initialize Lens Driver"
                    n182 = local read "Calibration"() -> (w359:T2)
                    n183 = for {
                      tunnel: w370 -> [w403]
                      tunnel: [w400] -> w362
                      tunnel: string[] ["Start", "MwDA", "CrMA00", "CrMB00", "CrUA00", "CrUB00", "CrLA00", "CrLB00", "PwTA\u0002Ð\u0001@"] -> [w398] mode=indexing
                      tunnel: [w397] -> w361
                      shift-right: [w401] -> w363
                      shift-left: w359 -> [w402]
                      shift-right: [w399] -> w364
                      shift-left: w371 -> [w404]
                      n184 = call "write read Lens Driver.vi"("VISA resource name"=w403, "command"=w398, "Calibration"=w402, "error in (no error)"=w404) -> ("VISA resource name out"=w400:refnum<visa-resource-name>, "Calibration 2"=w401:T2, "Data"=w397:string, "error out"=w399:errorcluster)  [unwired: 4 in, 4 out]
                    }
                    n185 = String Subset(string=w361, offset (0)=w367, length (rest)=w367) -> (substring=w365:string)
                    n186 = Type Cast(type=u16 0 ("length (rest)"), x=w365) -> (*(type *) &x=w360:u16)
                    n187 = local write "ID"(w360) -> ()
                    n188 = while {
                      tunnel: [w373] -> w369
                      tunnel: [w374] -> w368
                      tunnel: w364 -> [w379]
                      tunnel: w363 -> [w378]
                      tunnel: w362 -> [w377]
                      stop <- w372 stop-if-true
                      # "When Send command is true, Current Ch A is sent to the Lens Driver, in the correct format. If answer exists it is displayed in Data. The update rate of the while loop is 2ms."
                      n189 = Wait Until Next ms Multiple(millisecond multiple=u32 2) -> ()  [unwired: 1 out]
                      n190 = case shown="True" TRUE ("Send command") {
                        tunnel: [w381 w396] -> w373
                        tunnel: w379 -> [w381 w395]
                        tunnel: w378 -> [_ w386]
                        tunnel: w377 -> [w380 w394]
                        tunnel: [w380 w387] -> w374
                        frame False {
                        }
                        frame True {
                          n191 = Unbundle By Name(w386) -> ("Max Current A"=w385:dbl)
                          n192 = call "potencia a corriente.vi"("Max current A"=w385, "Potencia"="Potencia inicial lente derecho") -> ("Corriente"=w383:dbl)
                          n193 = To Word Integer(number=w383) -> (16bit integer=w393:i16)
                          n194 = Type Cast(x=w393) -> (*(type *) &x=w392:string)  [unwired: 1 in]
                          n195 = Concatenate Strings("Aw", w392) -> (w389:string)
                          n196 = local write "Command to Port"(w389) -> ()
                          n197 = call "write read Lens Driver.vi"("VISA resource name"=w394, "command"=w389, "Calibration"=w386, "error in (no error)"=w395) -> ("VISA resource name out"=w387:refnum<visa-resource-name>, "Calibration 2"=w391:T2, "OK"=w390:bool, "Data"=w388:string, "error out"=w396:errorcluster)  [unwired: 4 in, 3 out]
                          n198 = local write "VISA resource name out"(w387) -> ()
                          n199 = local write "Calibration 2"(w391) -> ()
                          n200 = local write "Data"(w388) -> ()
                          n201 = local write "OK"(w390) -> ()
                          "DPT INICIALES D" <- "Potencia inicial lente derecho"
                        }
                      }
                      n202 = local read "Parar adquisicion"() -> (w372:bool)
                    }
                  }
                  frame Error {
                  }
                }
                n203 = VISA Close(VISA resource name=w321, error in (no error)=w320) -> (error out=w323:errorcluster)
                n204 = call <vilib>:"Simple Error Handler.vi"("error in (no error)"=w323) -> ("error out"=→"error out 3":errorcluster)  [unwired: 4 in, 4 out]
                n205 = local read "VISA resource name 2"() -> (w340:string)
                n206 = call-poly "VISA Configure Serial Port"("VISA resource name"=w340, "timeout (10sec)"=u32 2000, "Enable Termination\nChar (T)"=FALSE ("Enable Termination\nChar (T)"), "baud rate (9600)"=u32 115200, "error in (no error)"="error in (no error) 4") -> ("VISA resource name out"=w344:refnum<visa-resource-name>, "error out"=w346:errorcluster)  [unwired: 9 in]
                n207 = property class="Instr"(reference=w344, error in=w346, "TermChar"=u8 10 ("Message Based Settings:Termination Character"), "ASRL End In"=w348, "ASRL End Out"=w349) -> (reference out=w345:refnum<visa-resource-name>, error out=w347:errorcluster)
                n208 = VISA Set I/O Buffer Size(VISA resource name=w345, error in (no error)=w347) -> (VISA resource name out=w351:refnum<visa-resource-name>, error out=w352:errorcluster)  [unwired: 2 in]
                n209 = VISA Flush I/O Buffer(VISA resource name=w351, error in (no error)=w352) -> (VISA resource name out=w354:refnum<visa-resource-name>, error out=w353:errorcluster)  [unwired: 1 in]
                n210 = case shown="No Error" w353 {
                  tunnel: w353 -> [w420 w460]
                  tunnel: w354 -> [w419 w461]
                  tunnel: [w418 w460] -> w317
                  tunnel: [w417 w461] -> w316
                  frame No Error {
                    w416 = 2 ("length (rest)")
                    # "Initialize Lens Driver"
                    n211 = local read "Calibration"() -> (w408:T2)
                    n212 = for {
                      tunnel: w419 -> [w458]
                      tunnel: [w455] -> w411
                      tunnel: string[] ["Start", "MwDA", "CrMA00", "CrMB00", "CrUA00", "CrUB00", "CrLA00", "CrLB00", "PwTA\u0002Ð\u0001@"] -> [w453] mode=indexing
                      tunnel: [w452] -> w410
                      shift-right: [w456] -> w412
                      shift-left: w408 -> [w457]
                      shift-right: [w454] -> w413
                      shift-left: w420 -> [w459]
                      n213 = call "write read Lens Driver.vi"("VISA resource name"=w458, "command"=w453, "Calibration"=w457, "error in (no error)"=w459) -> ("VISA resource name out"=w455:refnum<visa-resource-name>, "Calibration 2"=w456:T2, "Data"=w452:string, "error out"=w454:errorcluster)  [unwired: 4 in, 4 out]
                    }
                    n214 = String Subset(string=w410, offset (0)=w416, length (rest)=w416) -> (substring=w414:string)
                    n215 = Type Cast(type=u16 0 ("length (rest)"), x=w414) -> (*(type *) &x=w409:u16)
                    n216 = local write "ID"(w409) -> ()
                    n217 = while {
                      tunnel: [w422] -> w418
                      tunnel: [w423] -> w417
                      tunnel: w413 -> [w428]
                      tunnel: w412 -> [w427]
                      tunnel: w411 -> [w426]
                      stop <- w421 stop-if-true
                      # "When Send command is true, Current Ch A is sent to the Lens Driver, in the correct format. If answer exists it is displayed in Data. The update rate of the while loop is 2ms."
                      n218 = Wait Until Next ms Multiple(millisecond multiple=u32 2) -> ()  [unwired: 1 out]
                      n219 = case shown="True" TRUE ("Send command") {
                        tunnel: [w430 w451] -> w422
                        tunnel: w428 -> [w430 w450]
                        tunnel: w427 -> [_ w438]
                        tunnel: w426 -> [w429 w449]
                        tunnel: [w429 w439] -> w423
                        frame False {
                        }
                        frame True {
                          n220 = Unbundle By Name(w438) -> ("Max Current A"=w437:dbl)
                          n221 = Multiply(x=15.8, y="Potencia inicial lente izquierdo") -> (x*y=w435:dbl)
                          n222 = Add(x=-6.8, y=w435) -> (x+y=w433:dbl)
                          n223 = Divide(x=w433, y=w437) -> (x/y=w436:dbl)
                          n224 = Multiply(x=4096.0, y=w436) -> (x*y=w447:dbl)
                          n225 = To Word Integer(number=w447) -> (16bit integer=w446:i16)
                          n226 = Type Cast(x=w446) -> (*(type *) &x=w445:string)  [unwired: 1 in]
                          n227 = Concatenate Strings("Aw", w445) -> (w441:string)
                          n228 = local write "Command to Port"(w441) -> ()
                          n229 = call "write read Lens Driver.vi"("VISA resource name"=w449, "command"=w441, "Calibration"=w438, "error in (no error)"=w450) -> ("VISA resource name out"=w439:refnum<visa-resource-name>, "Calibration 2"=w443:T2, "OK"=w442:bool, "Data"=w440:string, "error out"=w451:errorcluster)  [unwired: 4 in, 3 out]
                          n230 = local write "VISA resource name out 2"(w439) -> ()
                          n231 = local write "Calibration 2"(w443) -> ()
                          n232 = local write "Data"(w440) -> ()
                          n233 = local write "OK"(w442) -> ()
                          "DPT INICIALES I" <- "Potencia inicial lente izquierdo"
                        }
                      }
                      n234 = local read "Parar adquisicion"() -> (w421:bool)
                    }
                  }
                  frame Error {
                  }
                }
                n235 = VISA Close(VISA resource name=w316, error in (no error)=w317) -> (error out=w319:errorcluster)
                n236 = call <vilib>:"Simple Error Handler.vi"("error in (no error)"=w319) -> ("error out"=→"error out 4":errorcluster)  [unwired: 4 in, 4 out]
              }
              frame 1 {
                # "Mensaje que pregunta si desea realizar el experimento\ncon un nuevo usuario o con el actual"
                # "Se vuelven 0 los valores del WL y de la potencia óptica y distancia"
                # "En esta opcion se activa el modo experimento"
                n237 = property on="Waveform length" class="WFChart (strict)"("History Data"=dbl[][] [[0.0]]) -> ()  [unwired: 2 in, 2 out]
                n238 = property on="Potencia Optica" class="WFChart (strict)"("History Data"=dbl[] [0.0]) -> ()  [unwired: 2 in, 2 out]
                n239 = Two Button Dialog(message="Con quien desea realizar los experimentos?", 1:"Nuevo voluntario" ("F button name (\"Cancel\")"), 2:"Voluntario actual" ("T button name (\"OK\")")) -> (T button?=w480:bool)
                n240 = flat-sequence {
                  tunnel: w480 -> [w493]
                  tunnel: [w492] -> w478
                  tunnel: w477 -> [w492]
                  tunnel: [w485] -> w465
                  tunnel: w464 -> [w485]
                  tunnel: [w503] -> w481
                  tunnel: [w505] -> w479
                  tunnel: w478 -> [w505]
                  tunnel: [w504] -> w475
                  tunnel: w474 -> [w504]
                  tunnel: [w502] -> w466
                  tunnel: w465 -> [w502]
                  tunnel: w481 -> [w517]
                  tunnel: w479 -> [w516]
                  tunnel: [w515] -> w476
                  tunnel: w475 -> [w514]
                  tunnel: [w513] -> w472
                  tunnel: [w512] -> w471
                  tunnel: [w511] -> w469
                  tunnel: [w510] -> w467
                  tunnel: w466 -> [w510]
                  tunnel: w472 -> [w566]
                  tunnel: w471 -> [w549]
                  tunnel: [w566] -> w470
                  tunnel: w469 -> [w552]
                  tunnel: [w542] -> w468
                  tunnel: w467 -> [w542]
                  tunnel: [w569] -> w473
                  tunnel: w470 -> [w569]
                  tunnel: w468 -> [w567]
                  frame #0 {
                    # "Se guardan los datos de un nuevo voluntario"
                    n241 = Not(x=w493) -> (.not. x?=w487:bool)
                    n242 = case shown="True" w487 {
                      tunnel: [w496 w501] -> w491
                      tunnel: [w495 w500] -> w490
                      tunnel: [w497 w499] -> w489
                      tunnel: [w494 w498] -> w488
                      frame False {
                        n243 = local read "Enfermedad visual"() -> (w496:string)
                        n244 = local read "Nombre"() -> (w497:string)
                        n245 = local read "Cedula"() -> (w494:string)
                        n246 = local read "Edad"() -> (w495:string)
                      }
                      frame True {
                        n247 = call "Registro voluntario"() -> ("Enfermedad visual"=w501:string, "Edad"=w500:string, "Cedula"=w498:string, "Nombre"=w499:string)  [unwired: 14 in, 2 out]
                      }
                    }
                    "Cedula" <- w488
                    "Nombre" <- w489
                    "Edad" <- w490
                    "Enfermedad visual" <- w491
                    n248 = local write "T button?"(FALSE ("T button?")) -> ()
                  }
                  frame #1 {
                    n249 = Two Button Dialog(message="Qué tipo de experimento desea realizar?", 1:"Nuevo Experimento" ("F button name (\"Cancel\")"), 2:"Experimento existente" ("T button name (\"OK\")")) -> (T button?=w506:bool)
                    n250 = Not(x=w506) -> (.not. x?=w503:bool)
                  }
                  frame #2 {
                    # "A partir de la seleccion del experimento, se obtiene la descripcion correspondiente que será guardada en el archivo"
                    n251 = case shown="False" w517 {
                      tunnel: w516 -> [w519 w537]
                      tunnel: [w519 w536] -> w515
                      tunnel: w514 -> [w521 w535]
                      tunnel: [w521 w534] -> w513
                      tunnel: [w522 w533] -> w512
                      tunnel: [w518 w532] -> w511
                      frame False {
                        n252 = call "Display Message to User"() -> ()  [unwired: 10 in, 2 out]
                        n253 = flat-sequence {
                          tunnel: [w523] -> w520
                          tunnel: w519 -> [w523]
                          tunnel: [w531] -> w522
                          tunnel: w521 -> [w530]
                          tunnel: ["Menu experimentos"] -> _
                          tunnel: w520 -> [w528]
                          tunnel: [w527] -> w518
                          frame #0 {
                            n254 = while {
                              stop <- w524 stop-if-true
                              # "El sistema se queda en el loop hasta que el usuario elija el experimento que desea realizar"
                              n255 = event shown="[0] \"Elegir menu Exp\": Value Change" {
                                selector: _ -> [_ _]
                                dyn-events: _ -> [_ _]
                                timeout: _ -> [_ _]
                                tunnel: [TRUE FALSE] -> w524
                                event "Elegir menu Exp": Value Change {
                                n256 = event-data() -> ()  [unwired: 1 in, 4 out]
                                }
                                event Timeout {
                                n257 = event-data() -> ()  [unwired: 1 in, 3 out]
                                }
                              }
                            }
                          }
                          frame #1 {
                            n258 = Index Array(array=w530, index="Menu experimentos") -> (element=w531:string)
                            n259 = Index Array(array=w528, index="Menu experimentos") -> (element=w527:string)
                          }
                        }
                        "Array" <- w519
                      }
                      frame True {
                        # "Se añade el nuevo experimento al menu de seleccion de experimentos"
                        # "Se guarda el nuevo experimento en el archivo que los contiene"
                        n260 = call "Nuevo experimento"() -> ("Descripcion"=w533:string, "Nombre"=w532:string)  [unwired: 16 in, 2 out]
                        n261 = Insert Into Array(array=w535, new element=w533) -> (w534:string[])  [unwired: 1 in]
                        n262 = Insert Into Array(array=w537, new element=w532) -> (w536:string[])  [unwired: 1 in]
                        n263 = property on="Menu experimentos" class="Ring (strict)"("Strings []"=w536) -> ()  [unwired: 2 in, 2 out]
                        n264 = Insert Into Array(array=string[] [], new element #1=w532, new element #2=w533) -> (w539:string[])  [unwired: 1 in]
                        n265 = call-poly <vilib>:"Write Delimited Spreadsheet.vi"("file path (dialog if empty)"=path "C:/Users/TGM1603/Documents/LabVIEW Data/Experimentos_realizados", "1D data"=w539, "append to file? (new file:F)"=TRUE) -> ()  [unwired: 11 in, 2 out]
                      }
                    }
                  }
                  frame #3 {
                    # "Se guardan los datos generales del experimento en el archivo de excel"
                    n266 = local read "Frecuencia muestreo"() -> (w544:i32)
                    n267 = local read "factor decimacion"() -> (w548:i32)
                    n268 = local read "Enfermedad visual"() -> (w551:string)
                    n269 = local read "Cedula"() -> (w553:string)
                    n270 = local read "Edad"() -> (w550:string)
                    n271 = local read "Nombre"() -> (w554:string)
                    n272 = Get Date/Time In Seconds() -> (seconds since 1Jan1904=w565:timestamp)
                    n273 = Path To String(path="Carpeta") -> (string=w561:string)
                    n274 = Format Date/Time String(time format string (%c)="_%d-%m-%y_%H-%M", seconds (now)=w565) -> (date/time string=w563:string)  [unwired: 1 in]
                    n275 = Number To Fractional String(number=w548, precision (6)=i16 0) -> (F-format string=w547:string)  [unwired: 2 in]
                    n276 = local read "Cedula"() -> (w557:string)
                    n277 = Number To Fractional String(number=w544, precision (6)=i16 0) -> (F-format string=w545:string)  [unwired: 2 in]
                    n278 = Concatenate Strings(w561, "\\" ("string"), w557, w563, "_" ("string"), w552, ".xlsx" ("string")) -> (w559:string)
                    n279 = String To Path(string=w559) -> (path=w558:path)
                    "path" <- w558
                    n280 = call "MS Office Report"("Path to Save Report"=w558, "Cedula"=w553, "decimacion"=w547, "Edad"=w550, "Enfermedad"=w551, "Exp_nombre"=w552, "Experimento"=w549, "freq"=w545, "Nombre"=w554) -> ()  [unwired: 17 in, 2 out]
                    "Nombre 2" <- w552
                  }
                  frame #4 {
                    n281 = while {
                      shift-right: [w571] -> _
                      shift-left: enum16{"Inicio", "Tomar datos", ""}."Inicio" -> [w573]
                      tunnel: w567 -> [w570]
                      stop <- w572 stop-if-true
                      n282 = case shown="\"Tomar datos\"" w573 {
                        tunnel: [w574 w585] -> w571
                        tunnel: w570 -> [_ w580]
                        frame "Inicio", Default {
                          # "Se chequea si el usuario ha presionado el boton de comenzar el experimento. Si no lo ha hecho, se queda en este estado (0).\n Cuando lo presiona, pasa al estado de adquirir datios (1) ."
                          n283 = Select(t=enum16{"Inicio", "Tomar datos", ""}."Tomar datos", s="Iniciar experimento", f=enum16{"Inicio", "Tomar datos", ""}."Inicio") -> (s? t:f=w574:enum16{"Inicio", "Tomar datos", ""})
                        }
                        frame "Tomar datos" {
                          n284 = flat-sequence {
                            tunnel: [w672] -> w584
                            tunnel: [w671] -> w583
                            tunnel: [w670] -> w582
                            tunnel: [w669] -> w581
                            tunnel: w580 -> [w664]
                            tunnel: [w647] -> w579
                            tunnel: [w629] -> w578
                            tunnel: w584 -> [w950]
                            tunnel: w583 -> [w949]
                            tunnel: w582 -> [w948]
                            tunnel: w581 -> [w947]
                            tunnel: w579 -> [w944]
                            tunnel: w578 -> [w945]
                            tunnel: [enum16{"Inicio", "Tomar datos", ""}."Inicio"] -> w585
                            frame #0 {
                              w590 = 10123 items=["Finite Samples"=10178, "Continuous Samples"=10123, "Hardware Timed Single Point"=12522] ("sample mode")
                              w594 = 10083 items=["Default"=-1, "RSE"=10083, "NRSE"=10078, "Differential"=10106, "Pseudodifferential"=12529] ("input terminal configuration")
                              w616 = u16 0 items=["None", "Last Bit", "TermChar", "Break"] ("Serial Settings:End Mode for Writes")
                              w617 = u16 2 items=["None", "Last Bit", "TermChar"] ("Serial Settings:End Mode for Reads")
                              w638 = u16 0 items=["None", "Last Bit", "TermChar", "Break"] ("Serial Settings:End Mode for Writes")
                              w639 = u16 2 items=["None", "Last Bit", "TermChar"] ("Serial Settings:End Mode for Reads")
                              w662 = 100  # max queue size
                              # "[9] Se unen en una sola matriz los vectores de tiempo, distancia, potencia derecha y potencia izquierda."
                              # "[9]"
                              # "[12] Se unen en una sola matriz, los vectores de  tiempo de la señal EMG, amplitud de la señal EMG, tiempo de potencia óptica, distancia, potencia óptica derecha y potencia óptica izquierda, en ese orden."
                              # "[8]"
                              # "[7]"
                              # "[6]"
                              # "[5]"
                              # "Se usan registros de desplazamiento para concatenar en un solo vector los datos que se obtienen en cada iteracion. Así en \n[1] Se guarda la potencia del lente derecho.\n[2] Por medio de variables locales, se guarda la distancia que se obtuvo en el bloque de distancia.\n[3]  Por medio de variables locales, se guarda la potencia del lente izquierdo que se obtuvo en el bloque de control de potencia del lente izquierdo.\n[4] Se guarda el tiempo actual.\n[5] Se pasa el vector de de potencia derecha a variable a string con 2 cifras significativas. \n[6] Se ajusta el vector del tiempo para que se muestre un tiempo relativo, es decir, en donde el primer dato sea 0 y en los demas se aumente un dt.  Además, se pasa el vector a variable a string con 5 cifras significativas.\n[7] Se pasa el vector de de distancia a variable a string con 0 cifras significativas. \n[8] Se pasa el vector de de potencia izquierda a variable a string con 2 cifras significativas."
                              # "En esta cola se guarda los datos de la señal EMG\nEn el bloque de adquisición los añade al adquirirlos y  en el de procesamiento los elimina al procesarlos ."
                              # "Initialize VISA port with correct parameters"
                              # "Initialize VISA port with correct parameters"
                              # "Close VISA port after program stop. Otherwise this port is blocked."
                              # "Se adquiere la señal del circuito de adquisicion, en donde se define la frecuencia de muestreo y el factor de decimacion.\n[1] Se inicializa el canal de adquisicion\n[2] Se ajusta el canal para que lea muestras continuas y apartir de estas prooduzca waveform data.\n[3]  Se obtiene los datos de la señal: la amplitud Y, el tiempo de inicio y el delta t.\n[4] Se decima el vector de amplitud. \n[5] Se usan registros de desplazamiento para concatenenar en un solo vector los datos de la amplitud que se obtienen en cada iteración. \n[6] Se obtiene el vector del tiempo."
                              # "[11] Los vectores de amplitud y tiempo se transforman a formato texto con 4 y 5 cifras significativas respectivamente y se unen para formar un vector de 2 columnas."
                              # "[9] Se ajusta el vector del tiempo para que se muestre un tiempo relativo, es decir, en donde el primer dato sea 0 y en los demas se aumente un dt. \n[10] Se extrae el primer elemento del vector ya que este siempre es 0 y no aporta información"
                              # "[12]"
                              # "[11]"
                              # "[10]"
                              # "[9]"
                              # "[8] Se guarda la fecha/hora en que se inicio el experimento"
                              # "[7] Se usan registros de desplazamiento para concatenar en un solo vector los datos del tiempo que se obtienen en cada iteracion."
                              # "[1]"
                              n285 = local read "error in (no error)"() -> (w634:errorcluster)
                              n286 = local read "VISA resource name"() -> (w633:string)
                              n287 = local read "VISA resource name 2"() -> (w612:string)
                              n288 = call-poly "VISA Configure Serial Port"("VISA resource name"=w633, "timeout (10sec)"=u32 2000, "Enable Termination\nChar (T)"=FALSE ("Enable Termination\nChar (T)"), "baud rate (9600)"=u32 115200, "error in (no error)"=w634) -> ("VISA resource name out"=w643:refnum<visa-resource-name>, "error out"=w641:errorcluster)  [unwired: 9 in]
                              n289 = call-poly "VISA Configure Serial Port"("VISA resource name"=w612, "timeout (10sec)"=u32 2000, "Enable Termination\nChar (T)"=FALSE ("Enable Termination\nChar (T)"), "baud rate (9600)"=u32 115200, "error in (no error)"="error in (no error) 5") -> ("VISA resource name out"=w621:refnum<visa-resource-name>, "error out"=w619:errorcluster)  [unwired: 9 in]
                              n290 = property class="Instr"(reference=w643, error in=w641, "TermChar"=u8 10 ("Message Based Settings:Termination Character"), "ASRL End In"=w639, "ASRL End Out"=w638) -> (reference out=w642:refnum<visa-resource-name>, error out=w640:errorcluster)
                              n291 = property class="Instr"(reference=w621, error in=w619, "TermChar"=u8 10 ("Message Based Settings:Termination Character"), "ASRL End In"=w617, "ASRL End Out"=w616) -> (reference out=w620:refnum<visa-resource-name>, error out=w618:errorcluster)
                              n292 = VISA Set I/O Buffer Size(VISA resource name=w642, error in (no error)=w640) -> (VISA resource name out=w636:refnum<visa-resource-name>, error out=w635:errorcluster)  [unwired: 2 in]
                              n293 = VISA Set I/O Buffer Size(VISA resource name=w620, error in (no error)=w618) -> (VISA resource name out=w614:refnum<visa-resource-name>, error out=w613:errorcluster)  [unwired: 2 in]
                              n294 = VISA Flush I/O Buffer(VISA resource name=w636, error in (no error)=w635) -> (VISA resource name out=w632:refnum<visa-resource-name>, error out=w631:errorcluster)  [unwired: 1 in]
                              n295 = call-poly <vilib>:"DAQmx Create Virtual Channel.vi"("input terminal configuration"=w594, "physical channels"=tag "Dev1/ai0") -> ("task out"=w593:refnum<k21>, "error out"=w592:errorcluster)  [unwired: 12 in]
                              n296 = VISA Flush I/O Buffer(VISA resource name=w614, error in (no error)=w613) -> (VISA resource name out=w610:refnum<visa-resource-name>, error out=w609:errorcluster)  [unwired: 1 in]
                              n297 = invoke on="Parar adquisicion" class="Bool (strict)" method="Reinit To Default"() -> ()  [unwired: 3 in, 3 out]
                              n298 = Obtain Queue(max queue size (-1, unlimited)=w662, element data type="Cola tipo 2") -> (queue out=w661:refnum<queue>)  [unwired: 3 in, 2 out]
                              n299 = Enqueue Element(queue=w664, element=0.0) -> (queue out=w666:refnum<queue>)  [unwired: 2 in, 2 out]
                              n300 = call-poly <vilib>:"DAQmx Timing.vi"("task/channels in"=w593, "sample mode"=w590, "samples per channel"=1000, "rate"=1000.0, "error in"=w592) -> ("task out"=w588:refnum<k21>, "error out"=w587:errorcluster)  [unwired: 9 in]
                              n301 = call <vilib>:"DAQmx Start Task.vi"("task/channels in"=w588, "error in"=w587) -> ("task out"=w685:refnum<k21>, "error out"=w686:errorcluster)  [unwired: 12 in]
                              n302 = local read "tamaño buffer"() -> (w684:i32)
                              n303 = case shown="No Error" w609 {
                                tunnel: w609 -> [w709 w766]
                                tunnel: w610 -> [w708 w767]
                                tunnel: [w707 w766] -> w599
                                tunnel: [w706 w767] -> w598
                                tunnel: [w696 dbl[] [-30.0]] -> _
                                frame No Error {
                                w705 = 2 ("length (rest)")
                                # "Bloque de control del izquierdo. Se explica en el caso 0 de visualziación general"
                                # "Initialize Lens Driver"
                                n304 = local read "Calibration"() -> (w697:T2)
                                n305 = for {
                                tunnel: w708 -> [w763]
                                tunnel: [w760] -> w700
                                tunnel: string[] ["Start", "MwDA", "CrMA00", "CrMB00", "CrUA00", "CrUB00", "CrLA00", "CrLB00", "PwTA\u0002Ð\u0001@"] -> [w758] mode=indexing
                                tunnel: [w757] -> w699
                                shift-right: [w761] -> w701
                                shift-left: w697 -> [w762]
                                shift-right: [w759] -> w702
                                shift-left: w709 -> [w764]
                                n306 = call "write read Lens Driver.vi"("VISA resource name"=w763, "command"=w758, "Calibration"=w762, "error in (no error)"=w764) -> ("VISA resource name out"=w760:refnum<visa-resource-name>, "Calibration 2"=w761:T2, "Data"=w757:string, "error out"=w759:errorcluster)  [unwired: 4 in, 4 out]
                                }
                                n307 = String Subset(string=w699, offset (0)=w705, length (rest)=w705) -> (substring=w703:string)
                                n308 = Type Cast(type=u16 0 ("length (rest)"), x=w703) -> (*(type *) &x=w698:u16)
                                n309 = local write "ID"(w698) -> ()
                                n310 = while {
                                tunnel: [w714] -> w707
                                tunnel: [w715] -> w706
                                tunnel: w702 -> [w720]
                                tunnel: w701 -> [w719]
                                tunnel: w700 -> [w718]
                                shift-right: [w711] -> w696
                                shift-left: _ -> [w712]
                                stop <- w713 stop-if-true
                                # "When Send command is true, Current Ch A is sent to the Lens Driver, in the correct format. If answer exists it is displayed in Data. The update rate of the while loop is 2ms."
                                n311 = case shown="True" TRUE ("Send command") {
                                tunnel: [w726 w749] -> w714
                                tunnel: w720 -> [w726 w748]
                                tunnel: w719 -> [_ w729]
                                tunnel: w718 -> [w725 w747]
                                tunnel: [w725 w740] -> w715
                                tunnel: [dbl[] [-20.0] w739] -> w711
                                tunnel: w712 -> [_ w738]
                                frame False {
                                }
                                frame True {
                                n312 = local read "Potencia inicial lente izquierdo"() -> (w737:dbl)
                                n313 = local read "DPT dif."() -> (w736:dbl)
                                n314 = Add(x=w736, y=w737) -> (x+y=w732:dbl)
                                n315 = Absolute Value(x=w732) -> (abs(x)=w734:dbl)
                                n316 = Greater Or Equal?(x=6.0, y=w734) -> (x >= y?=w733:bool)
                                n317 = case shown="False" w733 {
                                tunnel: w732 -> [w752 w756]
                                tunnel: [w750 w756] -> w730
                                frame False {
                                n318 = Greater Or Equal?(x=u16 0, y=w752) -> (x >= y?=w753:bool)
                                n319 = case shown="False" w753 {
                                tunnel: [i16 6 ("x") i16 -6 ("x")] -> w750
                                frame False {
                                }
                                frame True {
                                }
                                }
                                }
                                frame True {
                                }
                                }
                                "Potencia izquierdo" <- w730
                                n320 = Unbundle By Name(w729) -> ("Max Current A"=w728:dbl)
                                n321 = call "potencia a corriente.vi"("Max current A"=w728, "Potencia"=w730) -> ("Corriente"=w731:dbl)
                                n322 = To Word Integer(number=w731) -> (16bit integer=w746:i16)
                                n323 = Type Cast(x=w746) -> (*(type *) &x=w745:string)  [unwired: 1 in]
                                n324 = Concatenate Strings("Aw", w745) -> (w742:string)
                                n325 = local write "Command to Port"(w742) -> ()
                                n326 = call "write read Lens Driver.vi"("VISA resource name"=w747, "command"=w742, "Calibration"=w729, "error in (no error)"=w748) -> ("VISA resource name out"=w740:refnum<visa-resource-name>, "Calibration 2"=w744:T2, "OK"=w743:bool, "Data"=w741:string, "error out"=w749:errorcluster)  [unwired: 4 in, 3 out]
                                n327 = local write "VISA resource name 2"(w740) -> ()
                                n328 = local write "Calibration 2"(w744) -> ()
                                n329 = local write "Data"(w741) -> ()
                                n330 = local write "OK"(w743) -> ()
                                n331 = Build Array (concatenate)(w738, w730) -> (w739:dbl[])
                                }
                                }
                                n332 = Wait Until Next ms Multiple(millisecond multiple=u32 10) -> ()  [unwired: 1 out]
                                n333 = local read "Parar adquisicion"() -> (w713:bool)
                                n334 = event shown="[0] \"Restablecer Iniciales\": Value Change" {
                                selector: _ -> [_ _]
                                dyn-events: _ -> [_ _]
                                timeout: 100 -> [_ _]
                                event "Restablecer Iniciales": Value Change {
                                n335 = event-data() -> ()  [unwired: 1 in, 3 out]
                                n336 = local read "Potencia inicial lente izquierdo"() -> (w721:dbl)
                                n337 = local read "Potencia inicial lente derecho"() -> (w722:dbl)
                                n338 = local write "Potencia izquierdo"(w721) -> ()
                                n339 = local write "Potencia derecho"(w722) -> ()
                                n340 = local write "DPT dif."(0.0 ("DPT dif.")) -> ()
                                }
                                event Timeout {
                                n341 = event-data() -> ()  [unwired: 1 in, 3 out]
                                }
                                }
                                }
                                }
                                frame Error {
                                }
                              }
                              n342 = case shown="No Error" w631 {
                                tunnel: w631 -> [w787 w877]
                                tunnel: w632 -> [w786 w878]
                                tunnel: [w785 w877] -> w659
                                tunnel: [w784 w878] -> w658
                                tunnel: [w773 dbl[] [-1.0]] -> w651
                                tunnel: [w772 dbl[] [-30.0]] -> w603
                                tunnel: [w770 dbl[] [-30.0]] -> w606
                                frame No Error {
                                w783 = 2 ("length (rest)")
                                # "Bloque de control del lente derecho. Se explica en el caso 0 de visualziación general"
                                # "Initialize Lens Driver"
                                n343 = local read "Calibration"() -> (w775:T2)
                                n344 = for {
                                tunnel: w786 -> [w872]
                                tunnel: [w869] -> w778
                                tunnel: string[] ["Start", "MwDA", "CrMA00", "CrMB00", "CrUA00", "CrUB00", "CrLA00", "CrLB00", "PwTA\u0002Ð\u0001@"] -> [w867] mode=indexing
                                tunnel: [w866] -> w777
                                shift-right: [w870] -> w779
                                shift-left: w775 -> [w871]
                                shift-right: [w868] -> w780
                                shift-left: w787 -> [w873]
                                n345 = call "write read Lens Driver.vi"("VISA resource name"=w872, "command"=w867, "Calibration"=w871, "error in (no error)"=w873) -> ("VISA resource name out"=w869:refnum<visa-resource-name>, "Calibration 2"=w870:T2, "Data"=w866:string, "error out"=w868:errorcluster)  [unwired: 4 in, 4 out]
                                }
                                n346 = String Subset(string=w777, offset (0)=w783, length (rest)=w783) -> (substring=w781:string)
                                n347 = Type Cast(type=u16 0 ("length (rest)"), x=w781) -> (*(type *) &x=w776:u16)
                                n348 = local write "ID"(w776) -> ()
                                n349 = while {
                                tunnel: [w800] -> w785
                                tunnel: [w801] -> w784
                                tunnel: w780 -> [w806]
                                tunnel: w779 -> [w805]
                                tunnel: w778 -> [w804]
                                shift-right: [w793] -> w773
                                shift-left: dbl[] [0.0] -> [w794]
                                shift-right: [w788] -> w772
                                shift-left: dbl[] [0.0] -> [w798]
                                shift-right: [w791] -> w770
                                shift-left: dbl[] [0.0] -> [w790]
                                stop <- w799 stop-if-true
                                # "[4]"
                                # "[3]"
                                # "When Send command is true, Current Ch A is sent to the Lens Driver, in the correct format. If answer exists it is displayed in Data. The update rate of the while loop is 2ms."
                                n350 = Wait Until Next ms Multiple(millisecond multiple=u32 10) -> ()  [unwired: 1 out]
                                n351 = case shown="True" TRUE ("Send command") {
                                tunnel: [w813 w832] -> w800
                                tunnel: w806 -> [w813 w831]
                                tunnel: w805 -> [_ w816]
                                tunnel: w804 -> [w812 w830]
                                tunnel: [w812 w822] -> w801
                                tunnel: [dbl[] [-20.0] w821] -> w788
                                tunnel: w798 -> [_ w820]
                                frame False {
                                }
                                frame True {
                                # "[1]"
                                n352 = local read "number"() -> (w827:u32)
                                n353 = local read "Potencia inicial lente derecho"() -> (w819:dbl)
                                n354 = case shown="2" w827 {
                                tunnel: [w833 w842 w857] -> w818
                                tunnel: w819 -> [w835 w837 w852]
                                tunnel: w819 -> [_ w836 w851]
                                frame 0, Default {
                                n355 = local read "DPT dif."() -> (w834:dbl)
                                n356 = Add(x=w835, y=w834) -> (x+y=w833:dbl)
                                }
                                frame 1 {
                                n357 = local read "DPT dif."() -> (w838:dbl)
                                n358 = Add(x=w837, y=w838) -> (x+y=w839:dbl)
                                n359 = Less Or Equal?(x=w839, y=6.0) -> (x <= y?=w841:bool)
                                n360 = case shown="True" w841 {
                                tunnel: [w844 w848] -> w842
                                tunnel: w836 -> [w843 w847]
                                frame False {
                                n361 = local read "DPT dif."() -> (w845:dbl)
                                n362 = Add(x=w843, y=w845) -> (x+y=w844:dbl)
                                }
                                frame True {
                                n363 = local read "DPT dif."() -> (w849:dbl)
                                n364 = local read "Incremento"() -> (w846:dbl)
                                n365 = Add(x=w849, y=w846) -> (x+y=w850:dbl)
                                n366 = local write "DPT dif."(w850) -> ()
                                n367 = Add(x=w847, y=w850) -> (x+y=w848:dbl)
                                }
                                }
                                }
                                frame 2 {
                                n368 = local read "DPT dif."() -> (w856:dbl)
                                n369 = Add(x=w856, y=w852) -> (x+y=w853:dbl)
                                n370 = Greater Or Equal?(x=w853, y=-6.0) -> (x >= y?=w854:bool)
                                n371 = case shown="True" w854 {
                                tunnel: [w859 w863] -> w857
                                tunnel: w851 -> [w858 w862]
                                frame False {
                                n372 = local read "DPT dif."() -> (w860:dbl)
                                n373 = Add(x=w858, y=w860) -> (x+y=w859:dbl)
                                }
                                frame True {
                                n374 = local read "DPT dif."() -> (w865:dbl)
                                n375 = local read "Incremento"() -> (w861:dbl)
                                n376 = Subtract(x=w865, y=w861) -> (x-y=w864:dbl)
                                n377 = local write "DPT dif."(w864) -> ()
                                n378 = Add(x=w862, y=w864) -> (x+y=w863:dbl)
                                }
                                }
                                }
                                }
                                "Potencia derecho" <- w818
                                n379 = Unbundle By Name(w816) -> ("Max Current A"=w815:dbl)
                                n380 = call "potencia a corriente.vi"("Max current A"=w815, "Potencia"=w818) -> ("Corriente"=w817:dbl)
                                n381 = To Word Integer(number=w817) -> (16bit integer=w829:i16)
                                n382 = Type Cast(x=w829) -> (*(type *) &x=w828:string)  [unwired: 1 in]
                                n383 = Concatenate Strings("Aw", w828) -> (w824:string)
                                n384 = local write "Command to Port"(w824) -> ()
                                n385 = call "write read Lens Driver.vi"("VISA resource name"=w830, "command"=w824, "Calibration"=w816, "error in (no error)"=w831) -> ("VISA resource name out"=w822:refnum<visa-resource-name>, "Calibration 2"=w826:T2, "OK"=w825:bool, "Data"=w823:string, "error out"=w832:errorcluster)  [unwired: 4 in, 3 out]
                                n386 = local write "VISA resource name out"(w822) -> ()
                                n387 = local write "Calibration 2"(w826) -> ()
                                n388 = local write "Data"(w823) -> ()
                                n389 = local write "OK"(w825) -> ()
                                n390 = Build Array (concatenate)(w820, w818) -> (w821:dbl[])
                                }
                                }
                                "Potencia Optica" <- w788
                                n391 = local read "Parar adquisicion"() -> (w799:bool)
                                n392 = local read "Potencia izquierdo"() -> (w789:dbl)
                                n393 = property on="Potencia optica" class="WFChart (strict)"("YScale.ScaleFit"="Auto scale Y") -> ()  [unwired: 2 in, 2 out]
                                n394 = Get Date/Time In Seconds() -> (seconds since 1Jan1904=w795:timestamp)
                                n395 = To Double Precision Float(number=w795) -> (double precision float=w792:dbl)
                                n396 = property on="Potencia Optica" class="WFChart (strict)"("XScale.ScaleFit"="Auto scale X") -> ()  [unwired: 2 in, 2 out]
                                n397 = Build Array (concatenate)(w794, w792) -> (w793:dbl[])
                                n398 = case shown="0, Default" "Auto scale Y" {
                                frame 0, Default {
                                n399 = property on="Potencia Optica" class="WFChart (strict)"("YScale.Maximum"="Escala Y max") -> ()  [unwired: 2 in, 2 out]
                                n400 = property on="Potencia Optica" class="WFChart (strict)"("YScale.Minimum"="Escala Y min") -> ()  [unwired: 2 in, 2 out]
                                }
                                frame 1 {
                                }
                                }
                                n401 = Build Array (concatenate)(w790, w789) -> (w791:dbl[])
                                n402 = case shown="0, Default" "Auto scale X" {
                                frame 0, Default {
                                n403 = property on="Potencia Optica" class="WFChart (strict)"("XScale.Maximum"="Escala X max") -> ()  [unwired: 2 in, 2 out]
                                n404 = property on="Potencia Optica" class="WFChart (strict)"("XScale.Minimum"="Escala X min") -> ()  [unwired: 2 in, 2 out]
                                }
                                frame 1 {
                                }
                                }
                                }
                                }
                                frame Error {
                                }
                              }
                              n405 = while {
                                tunnel: w666 -> [w889]
                                shift-right: [w891] -> _
                                shift-left: dbl[] [0.0] -> [w897]
                                shift-right: [w890] -> _
                                shift-left: u32[] [0] -> [w892]
                                tunnel: [w889] -> _
                                tunnel: w661 -> [w881]
                                stop <- w880 stop-if-true
                                # "Bloque de procesamiento.  Se explica en el caso 0 de visualización general"
                                n406 = local read "WL"() -> (w888:dbl)
                                n407 = local read "Parar adquisicion"() -> (w880:bool)
                                n408 = local read "Limite superior WL"() -> (w885:dbl)
                                n409 = call "waveform_length.vi"("WL"=w888, "Cola WL"=w889, "Datos entrada"=w881) -> ("WL 2"=w896:dbl)
                                n410 = local read "Limite inferior WL"() -> (w887:dbl)
                                n411 = local write "WL"(w896) -> ()
                                n412 = Build Array (concatenate)(w897, w896) -> (w891:dbl[])
                                n413 = In Range and Coerce(upper limit=w885, x=w896, lower limit=w887) -> (In Range?=w894:bool)  [unwired: 1 out]
                                n414 = Greater?(x=w896, y=w885) -> (0:w895:bool)
                                n415 = local read "Escala autom. X"() -> (w882:u8)
                                n416 = local read "Escala autom. Y"() -> (w883:u8)
                                n417 = Build Array(w895, w894) -> (w893:bool[])
                                n418 = Boolean Array To Number(Boolean array=w893) -> (number=w886:u32)
                                n419 = local write "number"(w886) -> ()
                                n420 = Build Array (concatenate)(w892, w886) -> (w890:u32[])
                                n421 = Build Array(w891, w890) -> (w884:dbl[][])
                                n422 = Transpose 2D Array(2D array=w884) -> (transposed array=w879:dbl[][])
                                n423 = local write "Waveform length"(w879) -> ()
                                n424 = property on="Waveform length" class="WFChart (strict)"("XScale.ScaleFit"=w882) -> ()  [unwired: 2 in, 2 out]
                                n425 = property on="Waveform length" class="WFChart (strict)"("YScale.ScaleFit"=w883) -> ()  [unwired: 2 in, 2 out]
                                n426 = case shown="0, Default" w883 {
                                frame 0, Default {
                                n427 = local read "Maximo escala Y"() -> (w901:dbl)
                                n428 = local read "Minimo escala Y"() -> (w900:dbl)
                                n429 = property on="Waveform length" class="WFChart (strict)"("YScale.Maximum"=w901) -> ()  [unwired: 2 in, 2 out]
                                n430 = property on="Waveform length" class="WFChart (strict)"("YScale.Minimum"=w900) -> ()  [unwired: 2 in, 2 out]
                                }
                                frame 1 {
                                }
                                }
                                n431 = case shown="0, Default" w882 {
                                frame 0, Default {
                                n432 = local read "Minimo escala X"() -> (w899:dbl)
                                n433 = local read "Maximo escala X"() -> (w898:dbl)
                                n434 = property on="Waveform length" class="WFChart (strict)"("XScale.Minimum"=w899) -> ()  [unwired: 2 in, 2 out]
                                n435 = property on="Waveform length" class="WFChart (strict)"("XScale.Maximum"=w898) -> ()  [unwired: 2 in, 2 out]
                                }
                                frame 1 {
                                }
                                }
                              }
                              n436 = while {
                                tunnel: w685 -> [w934]
                                tunnel: w684 -> [w931]
                                tunnel: [w932] -> w674
                                shift-right: [w929] -> w673
                                shift-left: w686 -> [w933]
                                tunnel: [w924] -> w694
                                shift-right: [w923] -> w671
                                shift-left: _ -> [w922]
                                shift-right: [w913] -> w676
                                shift-left: dbl[] [0.0] -> [w918]
                                shift-right: [w914] -> w681
                                shift-left: dbl[] [0.0] -> [w915]
                                tunnel: w661 -> [w906]
                                i -> [w925]
                                stop <- w928 stop-if-true
                                w927 = 10.0  # timeout (s)
                                # "[7]"
                                # "[6]"
                                # "[5]"
                                # "[4]"
                                # "[3]"
                                # "[2]"
                                n437 = local read "Escala automatica X"() -> (w904:u8)
                                n438 = local read "Escala automatica Y"() -> (w903:u8)
                                n439 = property on="Senal EMG" class="WFGraph (strict)"("XScale.ScaleFit"=w904) -> ()  [unwired: 2 in, 2 out]
                                n440 = case shown="0, Default" w904 {
                                frame 0, Default {
                                n441 = local read "X Scale.Range:Increment"() -> (w937:dbl)
                                n442 = local read "X Scale.Range:Minimum"() -> (w938:dbl)
                                n443 = local read "X Scale.Range:Maximum"() -> (w939:dbl)
                                n444 = property on="Senal EMG" class="WFGraph (strict)"("XScale.Increment"=w937) -> ()  [unwired: 2 in, 2 out]
                                n445 = property on="Senal EMG" class="WFGraph (strict)"("XScale.Minimum"=w938) -> ()  [unwired: 2 in, 2 out]
                                n446 = property on="Senal EMG" class="WFGraph (strict)"("XScale.Maximum"=w939) -> ()  [unwired: 2 in, 2 out]
                                }
                                frame 1 {
                                }
                                }
                                n447 = local read "Parar adquisicion"() -> (w909:bool)
                                n448 = call-poly <vilib>:"DAQmx Read.vi"("task/channels in"=w934, "number of samples per channel"=w931, "timeout"=w927, "error in"=w933) -> ("task out"=w932:refnum<k21>, "data"=w919:waveform(dbl)[], "error out"=w929:errorcluster)  [unwired: 9 in]
                                n449 = Unbundle By Name(w929) -> ("status"=w930:bool)
                                n450 = Or(x=w930, y=w909) -> (x .or. y?=w928:bool)
                                n451 = property on="Senal EMG" class="WFGraph (strict)"("YScale.ScaleFit"=w903) -> ()  [unwired: 2 in, 2 out]
                                n452 = local write "Senal EMG"(w919) -> ()
                                n453 = case shown="0, Default" w903 {
                                frame 0, Default {
                                n454 = local read "Y Scale.Range:Maximum"() -> (w936:dbl)
                                n455 = local read "Y Scale.Range:Minimum"() -> (w935:dbl)
                                n456 = property on="Senal EMG" class="WFGraph (strict)"("YScale.Minimum"=w935) -> ()  [unwired: 2 in, 2 out]
                                n457 = property on="Senal EMG" class="WFGraph (strict)"("YScale.Maximum"=w936) -> ()  [unwired: 2 in, 2 out]
                                }
                                frame 1 {
                                }
                                }
                                n458 = call-poly <vilib>:"Index Waveform Array.vi"("index"=0, "waveform array"=w919) -> ("waveform"=w917:waveform(dbl))  [unwired: 8 in, 1 out]
                                n459 = Unbundle By Name(w917) -> ("Y"=w907:dbl[], "t0"=w924:timestamp)  [unwired: 1 out]
                                n460 = call-poly <vilib>:"Decimate (continuous).vi"("averaging"=TRUE, "decimating factor"="factor decimacion", "X"=w907) -> ("Decimated Array"=w902:dbl[])  [unwired: 7 in, 1 out]
                                n461 = Lossy Enqueue Element(queue=w906, element=w902) -> ()  [unwired: 1 in, 4 out]
                                n462 = Build Array (concatenate)(w918, w902) -> (w913:dbl[])
                                n463 = case shown="1" w925 {
                                tunnel: w924 -> [_ w943]
                                tunnel: [w941 w942] -> w923
                                tunnel: w922 -> [w941 _]
                                frame 0, Default {
                                }
                                frame 1 {
                                # "[8]"
                                n464 = Format Date/Time String(seconds (now)=w943) -> (date/time string=w942:string)  [unwired: 2 in]
                                }
                                }
                                n465 = local read "factor decimacion"() -> (w910:i32)
                                n466 = call-poly <vilib>:"Get Waveform Time Array.vi"("waveform in"=w917) -> ("X array"=w916:timestamp[])  [unwired: 9 in, 1 out]
                                n467 = event shown="[0] \"Ganancia\": Value Change" {
                                selector: _ -> [_ _]
                                dyn-events: _ -> [_ _]
                                timeout: 1 -> [_ _]
                                tunnel: "Ganancia" -> [w940 _]
                                event "Ganancia": Value Change {
                                n468 = event-data() -> ()  [unwired: 1 in, 4 out]
                                n469 = call "Ganancia programable.vi"("MOSI data"=w940) -> ()
                                }
                                event Timeout {
                                n470 = event-data() -> ()  [unwired: 1 in, 3 out]
                                }
                                }
                                n471 = To Double Precision Float(number=w916) -> (double precision float=w912:dbl[])
                                n472 = call-poly <vilib>:"Decimate (single shot).vi"("decimating factor"=w910, "X"=w912) -> ("Decimated Array"=w911:dbl[])  [unwired: 8 in, 1 out]
                                n473 = Build Array (concatenate)(w915, w911) -> (w914:dbl[])
                              }
                              n474 = call <vilib>:"DAQmx Clear Task.vi"("task in"=w674, "error in"=w673) -> ()  [unwired: 13 in, 1 out]
                              n475 = Index Array(array=w681, index=1) -> (element=w680:dbl)
                              n476 = Subtract(x=w681, y=w680) -> (x-y=w678:dbl[])
                              n477 = Delete From Array(array=w676, index=0) -> (array with subset deleted=w689:dbl[])  [unwired: 1 in, 1 out]
                              n478 = Delete From Array(array=w678, index=0) -> (array with subset deleted=w688:dbl[])  [unwired: 1 in, 1 out]
                              n479 = local read "path"() -> (w672:path)
                              n480 = Format Date/Time String(seconds (now)=w694) -> (date/time string=w670:string)  [unwired: 2 in]
                              n481 = Number To Fractional String(use system decimal point (T)=FALSE, number=w689, precision (6)=i16 4) -> (F-format string=w627:string[])  [unwired: 1 in]
                              n482 = Number To Fractional String(use system decimal point (T)=FALSE, number=w688, precision (6)=i16 5) -> (F-format string=w628:string[])  [unwired: 1 in]
                              n483 = Build Array(w628, w627) -> (w687:string[][])
                              n484 = Transpose 2D Array(2D array=w687) -> (transposed array=w669:string[][])
                              n485 = Delete From Array(array=w603, index=0) -> (array with subset deleted=w602:dbl[])  [unwired: 1 in, 1 out]
                              n486 = Index Array(array=w651, index=1) -> (element=w656:dbl)
                              n487 = Delete From Array(array=w606, index=0) -> (array with subset deleted=w605:dbl[])  [unwired: 1 in, 1 out]
                              n488 = VISA Close(VISA resource name=w598, error in (no error)=w599) -> (error out=w597:errorcluster)
                              n489 = Subtract(x=w651, y=w656) -> (x-y=w650:dbl[])
                              n490 = Number To Fractional String(use system decimal point (T)=FALSE, number=w602, precision (6)=i16 2) -> (F-format string=w625:string[])  [unwired: 1 in]
                              n491 = VISA Close(VISA resource name=w658, error in (no error)=w659) -> (error out=w660:errorcluster)
                              n492 = call <vilib>:"Simple Error Handler.vi"("error in (no error)"=w597) -> ("error out"=w596:errorcluster)  [unwired: 4 in, 4 out]
                              n493 = Delete From Array(array=w650, index=0) -> (array with subset deleted=w655:dbl[])  [unwired: 1 in, 1 out]
                              n494 = call <vilib>:"Simple Error Handler.vi"("error in (no error)"=w660) -> ("error out"=w657:errorcluster)  [unwired: 4 in, 4 out]
                              n495 = Number To Fractional String(use system decimal point (T)=FALSE, number=w605, precision (6)=i16 2) -> (F-format string=w586:string[])  [unwired: 1 in]
                              n496 = local write "error out"(w657) -> ()
                              n497 = local write "error out"(w596) -> ()
                              n498 = Number To Fractional String(use system decimal point (T)=FALSE, number=w655, precision (6)=i16 5) -> (F-format string=w626:string[])  [unwired: 1 in]
                              n499 = Build Array(w628, w627, w626, w586, w625) -> (w600:string[][])
                              n500 = Transpose 2D Array(2D array=w600) -> (transposed array=w629:string[][])
                              n501 = Build Array(w626, w586, w625) -> (w647:string[][])
                            }
                            frame #1 {
                              # "[13]"
                              # "[13] En esta case structure, se decide que datos se van a guardar. Esto lo hace el SUBVI llamado guardar datos de amplitud y tiempo."
                              n502 = Transpose 2D Array(2D array=w944) -> (transposed array=w946:string[][])
                              n503 = call <vilib>:"Three Button Dialog.vi"("Right Button Text (\"Cancel\")"="Señal EMG, potencia optica y distancia" ("Right Button Text (\"Cancel\")"), "Center Button Text (\"No\")"="Potencia optica" ("Center Button Text (\"No\")"), "Left Button Text (\"Yes\")"="Señal EMG" ("Left Button Text (\"Yes\")"), "message"="Elija que datos desea guardar") -> ("Which Button?"=w951:T3)  [unwired: 7 in]
                              n504 = case shown="\"Center Button\"" w951 {
                                tunnel: w950 -> [w960 w965 w968]
                                tunnel: w949 -> [w959 w964 w969]
                                tunnel: w948 -> [w958 w963 w970]
                                tunnel: w947 -> [w957 _ _]
                                tunnel: w946 -> [_ w962 _]
                                tunnel: w945 -> [_ _ w966]
                                frame "Left Button", Default {
                                # "Se guarda solo la señal EMG y su tiempo de adquisición."
                                n505 = call "Guardar datos de Amplitud y Tiempo.vi"("path"=w960, "Hora inicio"=w959, "Hora fin"=w958, "Datos experimento"=w957, "column headers"=string[] ["Tiempo(s)", "Amplitud(V)"]) -> ()  [unwired: 1 in]
                                }
                                frame "Center Button" {
                                # "Se guarda la potenica del lente derecho, del lente izquierdo, la distancia y el tiempo de estas variables."
                                n506 = call "Guardar datos de Amplitud y Tiempo.vi"("path"=w965, "Hora inicio"=w964, "Hora fin"=w963, "Datos experimento"=w962, "column headers"=string[] ["Tiempo(s)", "Distancia (cm)", "Potencia Optica derecho", "Potencia optica izquierdo"]) -> ()  [unwired: 1 in]
                                }
                                frame "Right Button" {
                                # "Se guarda el tiempo de adquisición así como la amplitud de la señal EMG,  la potenica del lente derecho, del lente izquierdo, la distancia y el tiempo de estas variables."
                                n507 = call "Guardar datos de Amplitud y Tiempo.vi"("path"=w968, "Hora inicio"=w969, "Hora fin"=w970, "Datos experimento"=w966, "column headers"=string[] ["Tiempo EMG(s)", "Amplitud(V)", "Tiempo DPT(s)", "Distancia (cm)", "Potencia optica derecho", "Potencia optica izquierdo"]) -> ()  [unwired: 1 in]
                                }
                              }
                            }
                            frame #2 {
                              # "Si el usuario desea repetir el experimento se vuelve al estado inicio en donde se espera que comience el experimento. De lo contrario se sale del loop y vuelve al menu principal."
                              n508 = Two Button Dialog(message="¿Desea repetir el experimento?", 1:"No" ("F button name (\"Cancel\")"), 2:"Si" ("T button name (\"OK\")")) -> (T button?=w973:bool)
                              n509 = Not(x=w973) -> (.not. x?=→"T button?":bool)
                            }
                          }
                        }
                      }
                      n510 = local read "T button?"() -> (w572:bool)
                    }
                  }
                }
                "Array 2" <- w477
              }
            }
          }
          event Timeout {
            n511 = event-data() -> ()  [unwired: 1 in, 3 out]
          }
        }
        "Array 3" <- w31
      }
      "Array 4" <- w22
    }
  }
